vi "Orbitron2Websdr_MainApp.vi"() -> ()   [LabVIEW 2021]
uses:
  Multitrack.llb/Window Rectangle.ctl
  <vilib>/Utility/error.llb/whitespace.ctl
  <vilib>/Utility/error.llb/DialogType.ctl
  <vilib>/Platform/TimedLoop/XDataNode/timing_clust.ctl
  <vilib>/Platform/TimedLoop/XDataNode/nitl_modes.ctl
  <vilib>/Platform/TimedLoop/XDataNode/wakeup.ctl
  <vilib>/Utility/inputDevices.llb/mouseAcquire.vi
  <vilib>/Utility/inputDevices.llb/closeMouse.vi
  <vilib>/Platform/TimedLoop/XDataNode/XDataNode.xnode
  <vilib>/Platform/TimedLoop/XDataNode/XDNodeRunTimeDep.lvlib
  <vilib>/Platform/browser.llb/Open URL in Default Browser (string).vi
panel:
  out "error out 3":errorcluster
  out "error out 2":errorcluster
  out "path 3":path
  in  "Tab Control":T1(tab)
  out "Click":bool
  in  "Lisa":string
  in  "load":bool
  in  "preferences":bool
  in  "cw":bool
  in  "WebPages":u16(ring)=2 items=["IJsselstein, the Netherlands, JO22MA62KJ.", "IS0GRB VHF WebSDR Receiver IS0GRB / south sartinian iland", "Novovoronezh WebSDR WX", "Nürnberg Skyscraper", "Goonhilly Earth Station"]
  in  "Truncate Left digits":i32 caption="kHz"
  in  "processes Box":string(combo)="WebSDR on R3KEE in Novovoronezh - Google Chrome"
  in  "Downlink Freq. Man.":dbl=137100.0 caption="kHz" format="%#_6f"
  in  "ManualLatch":bool
  in  "Radio Mode":bool=TRUE
  in  "Downlink corr.":dbl(knob) scale=-4.0..4.0
  in  "USB":bool
  in  "DeleteWebSDR":bool
  out "Satellite Name":string
  in  "FocusCheck":bool
  in  "Start browser":bool
  in  "Stop_Button":bool
  out "Title 2":string="WebSDR Cat Control"
  in  "FocusWebSDR":bool
  in  "OpenWebSDR":bool
  in  "AddWebSDR":bool
  in  "Stop Cat Control":bool
  in  "Cat Control":bool
  in  "TaskList_Button":bool
  out "Azimuth":string caption="°"
  out "Elevation":string caption="°"
  out "Downlink Freq.":string caption="KHz"
  in  "Type of DN":string
  in  "LSB":bool
  in  "AM":bool
  in  "FM":bool
  in  "EditWebSDR":bool
  out "Mode":string="Radio Manual mode"
  in  "ZoomOut":bool
  in  "ZoomIn":bool
  out "left":i16
  out "right":i16
  out "bottom":i16
  out "top":i16
  out "OverBrowser":bool
  out "MaOps":bool
  in  "Rate 2":i32(slide)=1 min=-10 max=10 scale=-10.0..10.0
  in  "Volume 2":i32(slide)=39 min=0 max=100 scale=0.0..100.0
  in  "TTS Voice":u16(ring)=1 items=["Microsoft Hedda Desktop - German", "Microsoft Zira Desktop - English (United States)"]
  in  "Output Device":u16(ring) items=["Lautsprecher (Realtek(R) Audio)", "CABLE Input (VB-Audio Virtual Cable)"]
  in  "Path of the webbrowser to start WebSDR":path=path "C:/Program Files/Google/Chrome/Application/chrome.exe"
  in  "goback_button":bool
  in  "Cancel Edit 2":bool
  out "data":string caption="DDE Message"
  in  "Sampling interval":u32=1000 caption="[ms]"
  in  "Load_button":bool
  in  "Cancel load":bool
  in  "Load controlfile":path=path "C:/Users/Setup/Documents/LabVIEW 2021"
  in  "Downlink corr.":string="0,000000"
  in  "Title":string="Add a new WebSDR database item"
  in  "Cancel Edit":bool
  in  "Edit_Button":bool
  in  "WebSDR Location / Name":string="Novovoronezh WebSDR WX"
  in  "Cancel Add":bool
  in  "Add_Button":bool
  in  "WebSDR URL":string="http://websdr.vrn.ru:8901/"
  in  "Window title":string="WebSDR on R3KEE in Novovoronezh - Google Chrome"
  in  "Truncate digits":string="2"
  out "Title 3":string="WebSDR Cat Control"
  in  "WebSDRDB":string[][](array[string])=[["IJsselstein, the Netherlands, JO22MA62KJ.", "WebSDR on Gerbrandy Tower in IJsselstein, NL - Google Chrome", "http://websdr.pi1utr.ampr.org:8901/", "0"], ["IS0GRB VHF WebSDR Receiver IS0GRB / south sartinian iland", "IS0GRB VHF WebSDR Receiver - Google Chrome", "http://websdr.is0grb.it:8902/", "2"], ["Novovoronezh WebSDR WX", "WebSDR on R3KEE in Novovoronezh - Google Chrome", "http://websdr.vrn.ru:8901/", "2"]]
  in  "Numeric":i32
  out "error out":errorcluster={"status"=FALSE, "code"=0, "source"="Get Window ID.vi"}
  out "Active Processses":string
  out "standard error":string
  out "standard output":string
  out "window rect 2":T2={"left"=-5, "top"=-564, "right"=1089, "bottom"=-2}
  in  "window names":string[](array[string])=["Orbitron 3.71", "WebSDR on R3KEE in Novovoronezh - Google Chrome", "Mydde", "RX-SSTV", "Task-Manager", "Einstellungen", "Einstellungen", "VIPM Service", "Microsoft Text Input Application", "Mail", "Posteingang – Hotmail ?- Mail", "Orbitron2Websdr_Win10Build", "RX-SSTV", "Program Manager", "LabVIEW"]
  in  "kill":bool
  in  "StopCatProgramatically":bool
  out "shutdown in":bool
  in  "iterCompleted":bool
  in  "slave4Killed":bool
  in  "slave3Killed":bool
  in  "slave1Killed":bool
  out "Elapsed Time (s)":dbl=3.000234603881836
  out "path 2":path
  out "path 4":path=path "C:/Users/Setup/Documents/LabVIEW 2021/Orbitron2Websdr_MainApp_20032021.ctr"
  out "path":path=path "C:/Users/Setup/Documents/LabVIEW 2021/Orbitron2Websdr_MainApp_20032021.ctr"
  out "concatenated string":string="Orbitron2Websdr_MainApp_20032021\\"
  out "string":string="C:\\Users\\Setup\\Documents\\LabVIEW 2021\\Orbitron2Websdr_MainApp_20032021.ctr"
  out "Parent Directory (+ Relative)":path=path "C:/Users/Setup/Documents/LabVIEW 2021"
  in  "dont write":bool
  in  "Interrupt":bool
  in  "AppName":string="WebSDR1"
  # "For Orbitron 3.71 MyDDE-Driver"
  # "To start WebSDR, you need a Webbrowser. We had good experiences using Firefox, so we selected Firefox as the default browser. If you want to start your WebSDR sessions with another browser,just select the executable of your preferred browser here:"
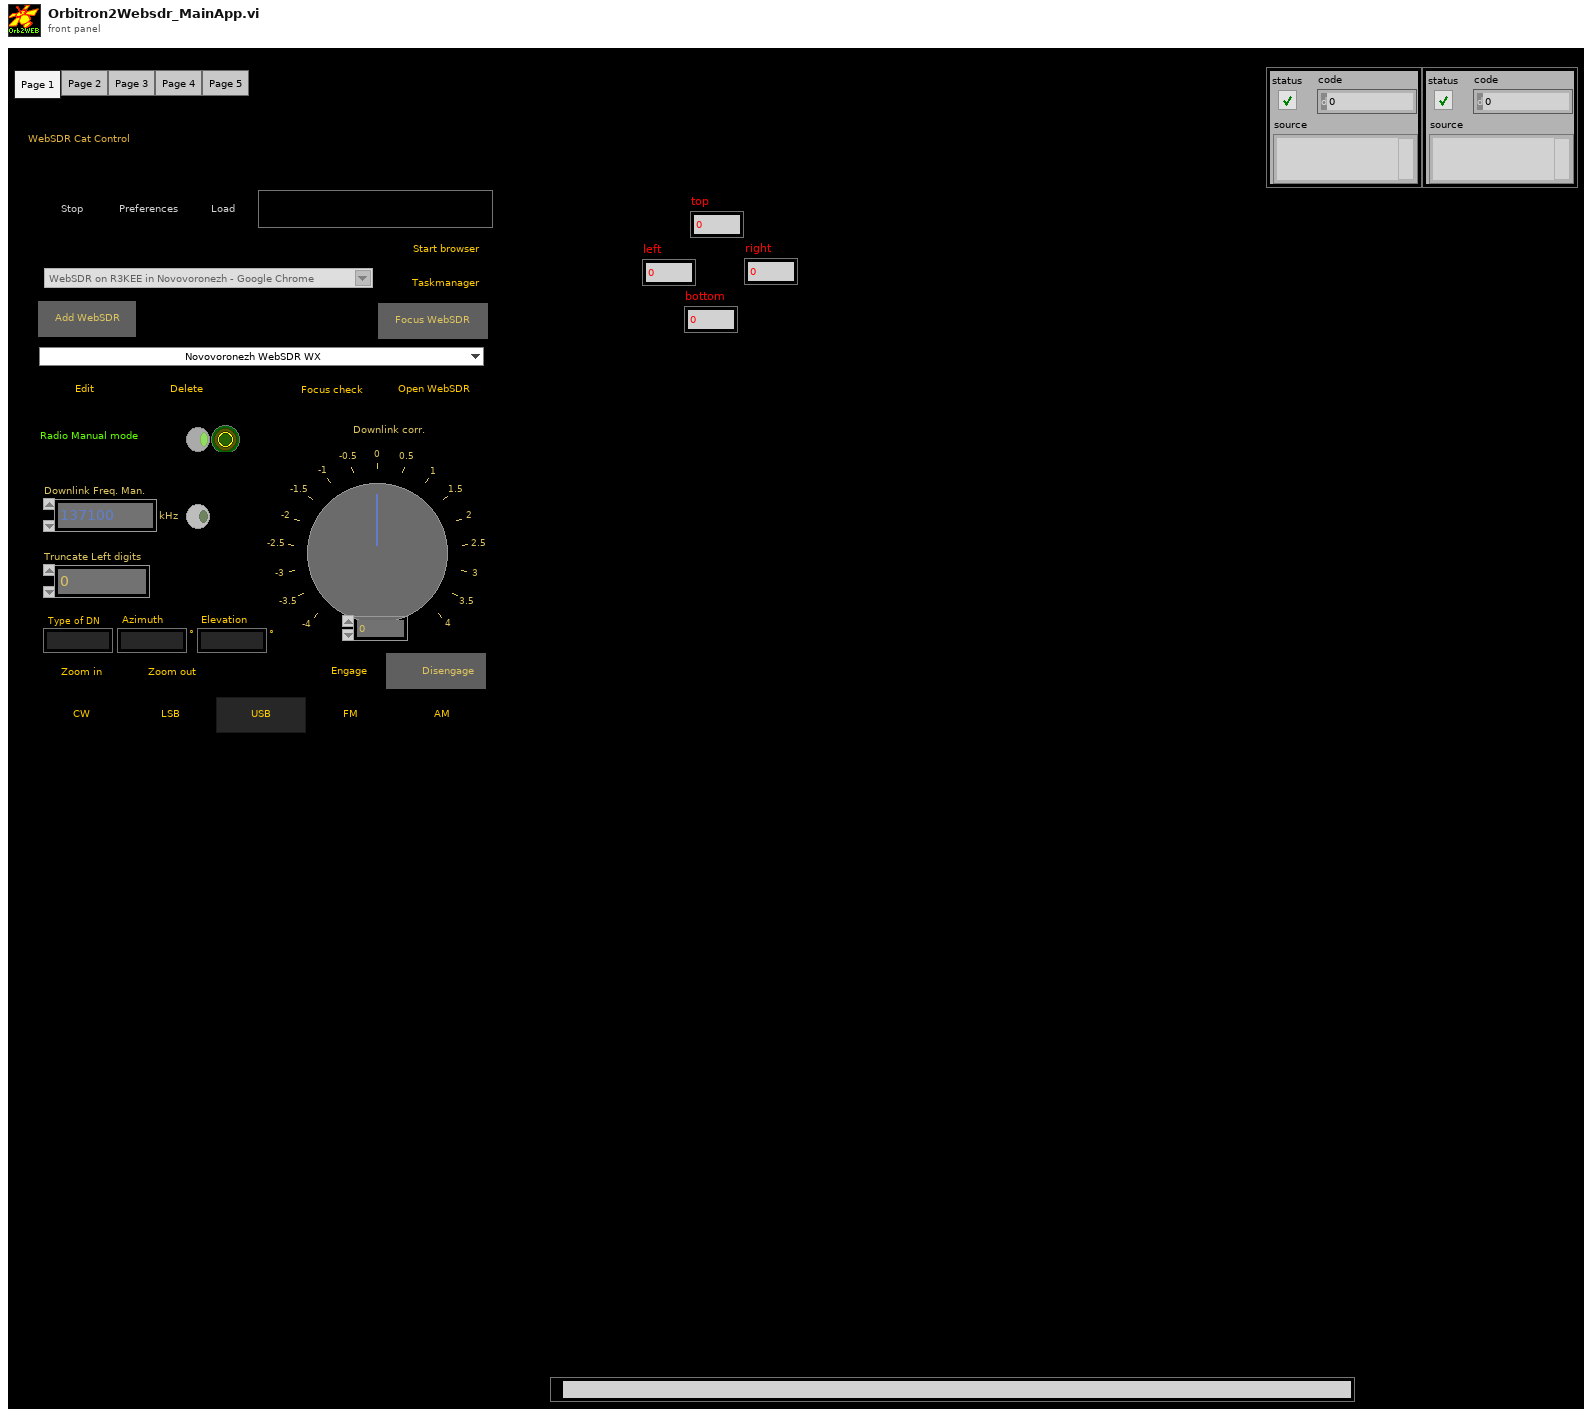
[diagram p1: front panel]
types:
  T1 = enum32{"Page 1", "Page 2", "Page 3", "Page 4", "Page 5"}
  T2 = typedef "Window Rectangle.ctl" = cluster{"left":i16, "top":i16, "right":i16, "bottom":i16}
  T3 = cluster{"Horizontal":i32, "Vertical":i32, "Scrolling":i32}
  T4 = cluster{"button 1":bool, "button 2":bool, "button 3":bool, "button 4":bool}
  T5 = typedef "DialogType.ctl" = u16
  T6 = enum8{"Enabled", "Disabled", "Disabled and Grayed Out"}
  T7 = enum16{"Get Number of Tasks", "Get Window Info", "Get Window Names"}
  T8 = cluster{"number of windows":i32, "total names length":u32, "number of tasks found":i32, "window handles":u32[], "process ID":u32}
  T9 = typedef "Window Refnum" = refnum<k1>
  T10 = typedef "XDNodeRunTimeDep.lvlib/timing_clust.ctl" = cluster{"Expected End [f-1]":u64, "Actual End [f-1]":u64, "Finished Late? [f-1]":bool, "Expected End [i-1]":u64, "Actual End [i-1]":u64, "Finished Late? [i-1]":bool, "Expected Start [i]":u64, "Actual Start [i]":u64, "Expected Start [f]":u64, "Actual Start [f]":u64, "Source Name":string, "Structure Name":string, "Period":i64, "Deadline":i64, "Offset":i64, "Start":i64, "Priority":i32, "Timeout":i32, "Mode":T11, "Wakeup Reason":T12, "Error":errorcluster, "Source Type":string, "Secondary Source Type":string, "Global End Time":u64, "Global Start Time":u64, "Frame Duration":u64, "Iteration Duration":u64, "Assigned CPU":i32, "I/O Scan Engine Mode":u32}
  T11 = typedef "XDNodeRunTimeDep.lvlib/nitl_modes.ctl" = enum32{"No Change", "Process missed periods, maintain original phase", "Discard missed periods, maintain original phase", "Process missed periods, ignore original phase", "Discard missed periods, ignore original phase"}
  T12 = typedef "XDNodeRunTimeDep.lvlib/wakeup.ctl" = enum32{"Normal", "Aborted", "Asynchronous wakeup", "Timing source error", "Timed loop error", "Timeout"}
  T13 = typedef "whitespace.ctl" = u16
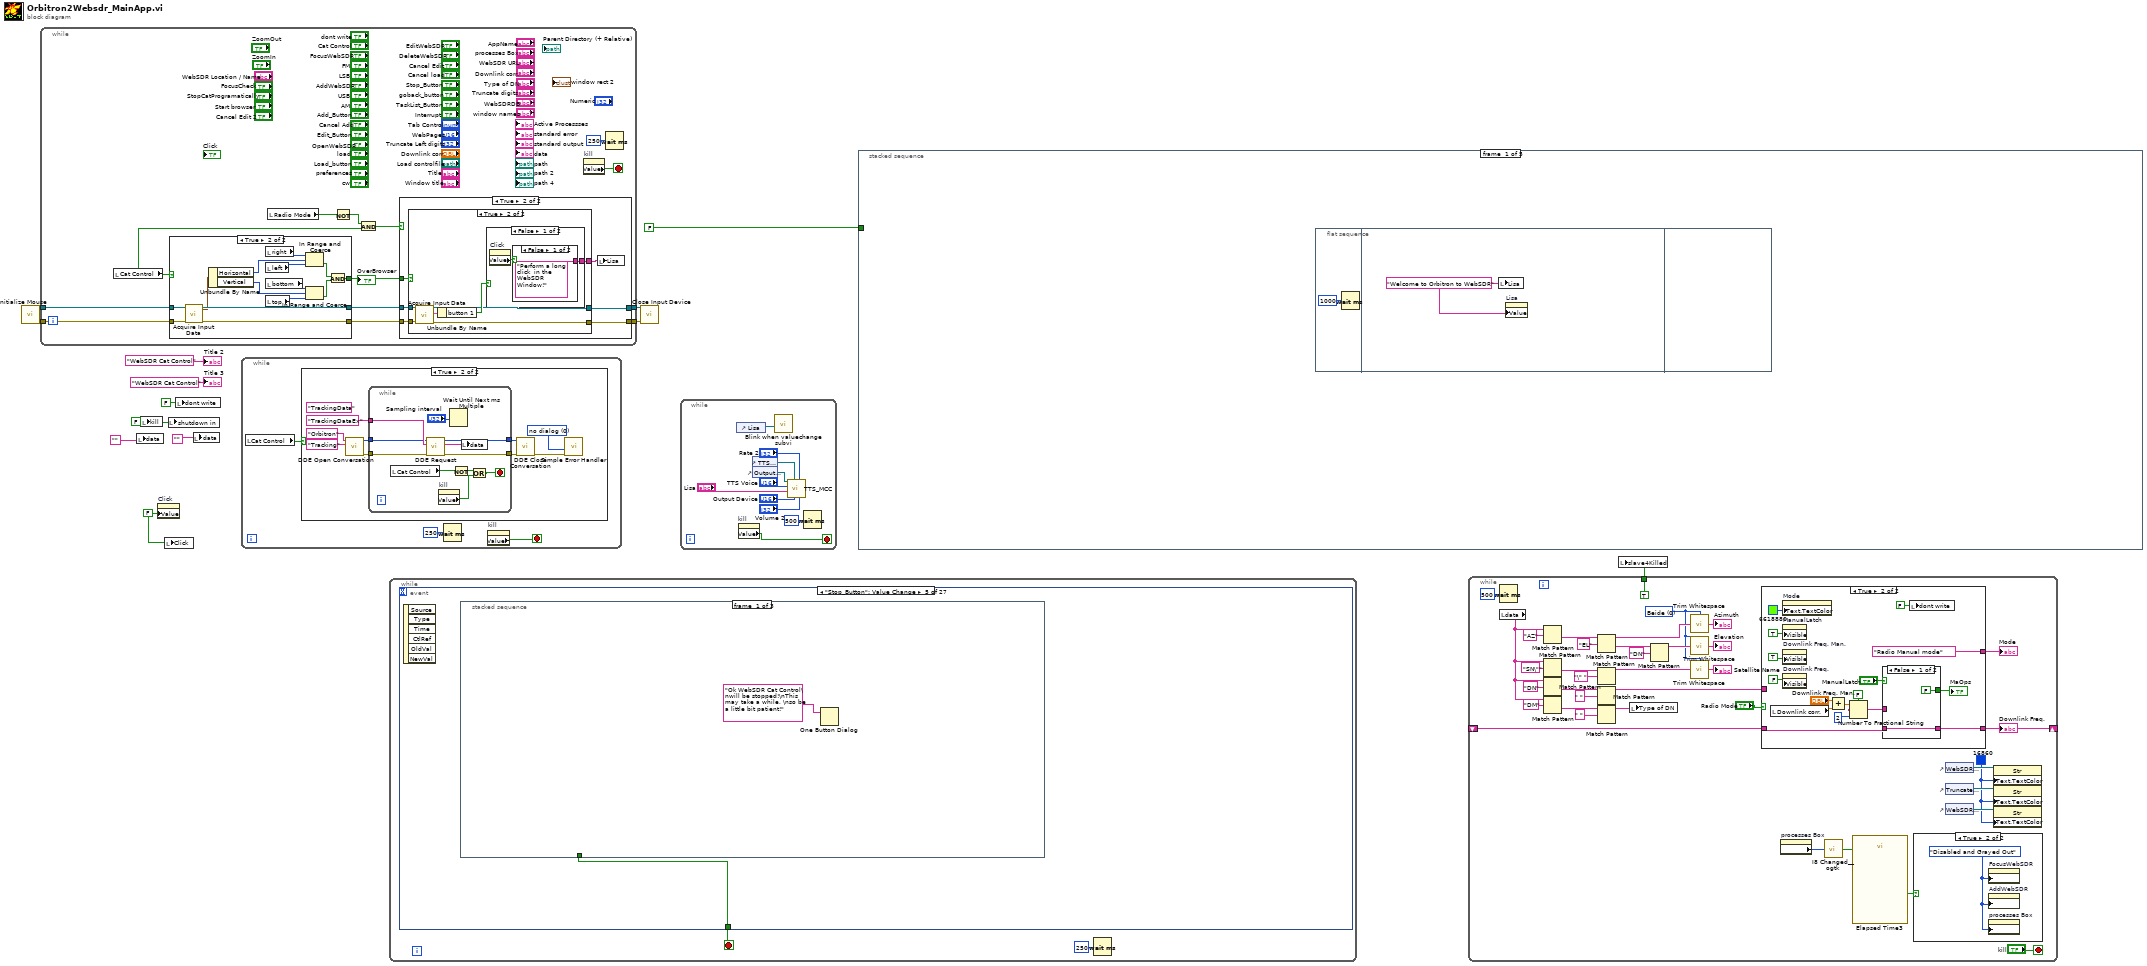
[diagram p0: block diagram]
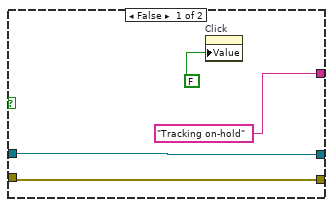
[diagram p3: hidden frame]
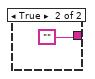
[diagram p4: hidden frame]
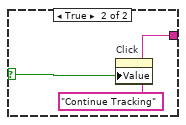
[diagram p5: hidden frame]
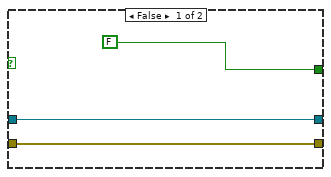
[diagram p6: hidden frame]
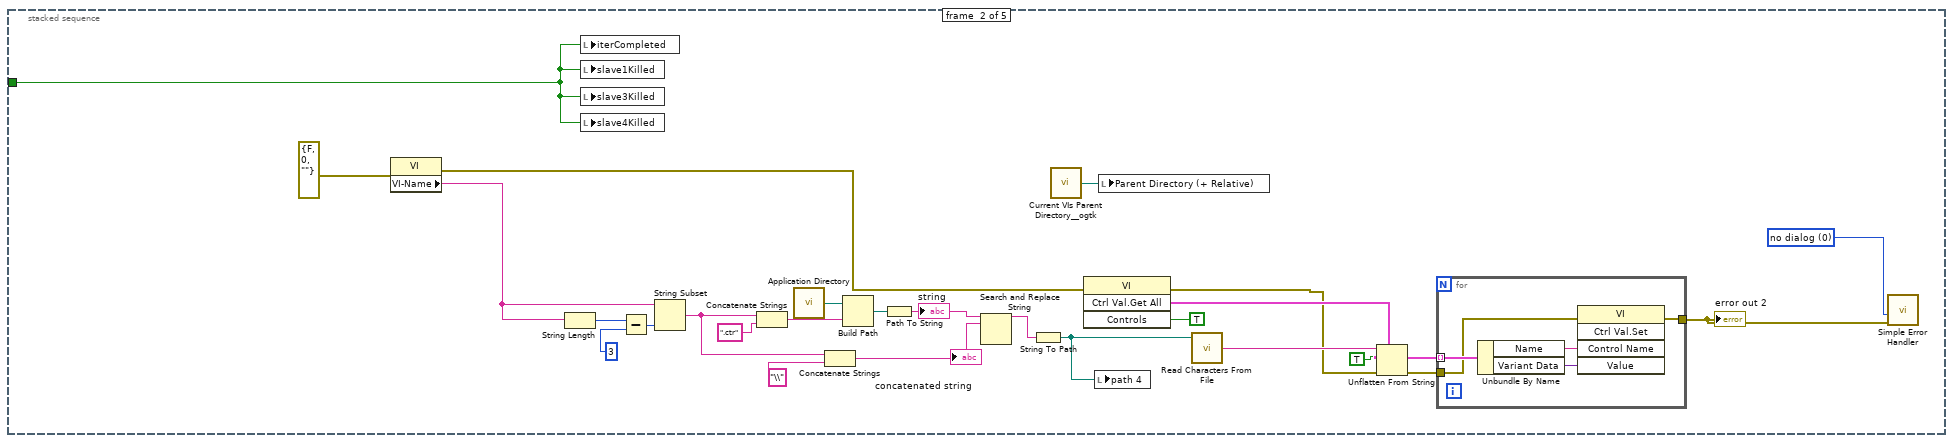
[diagram p8: hidden frame]
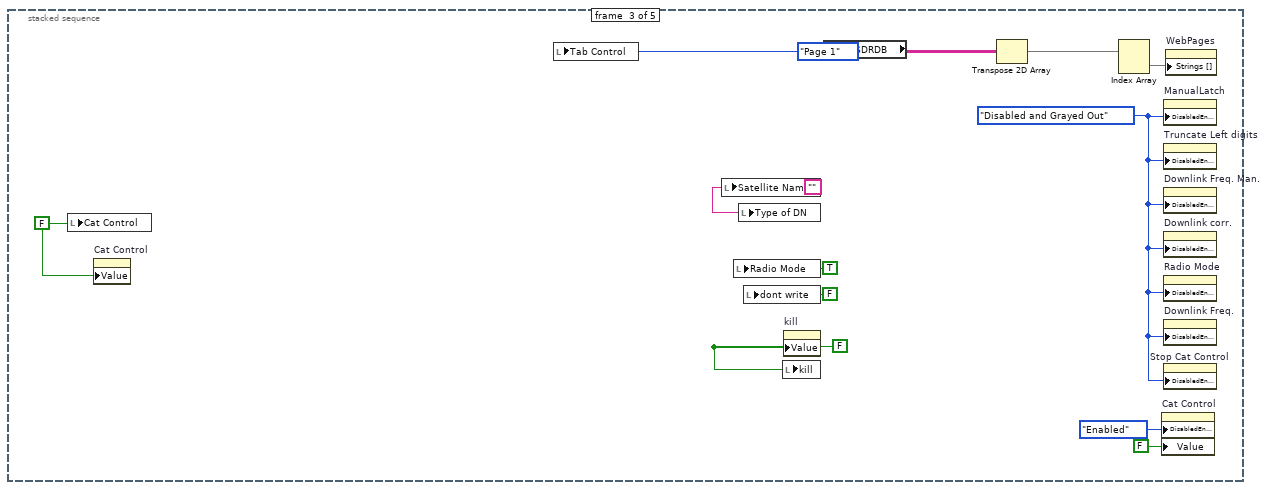
[diagram p9: hidden frame]
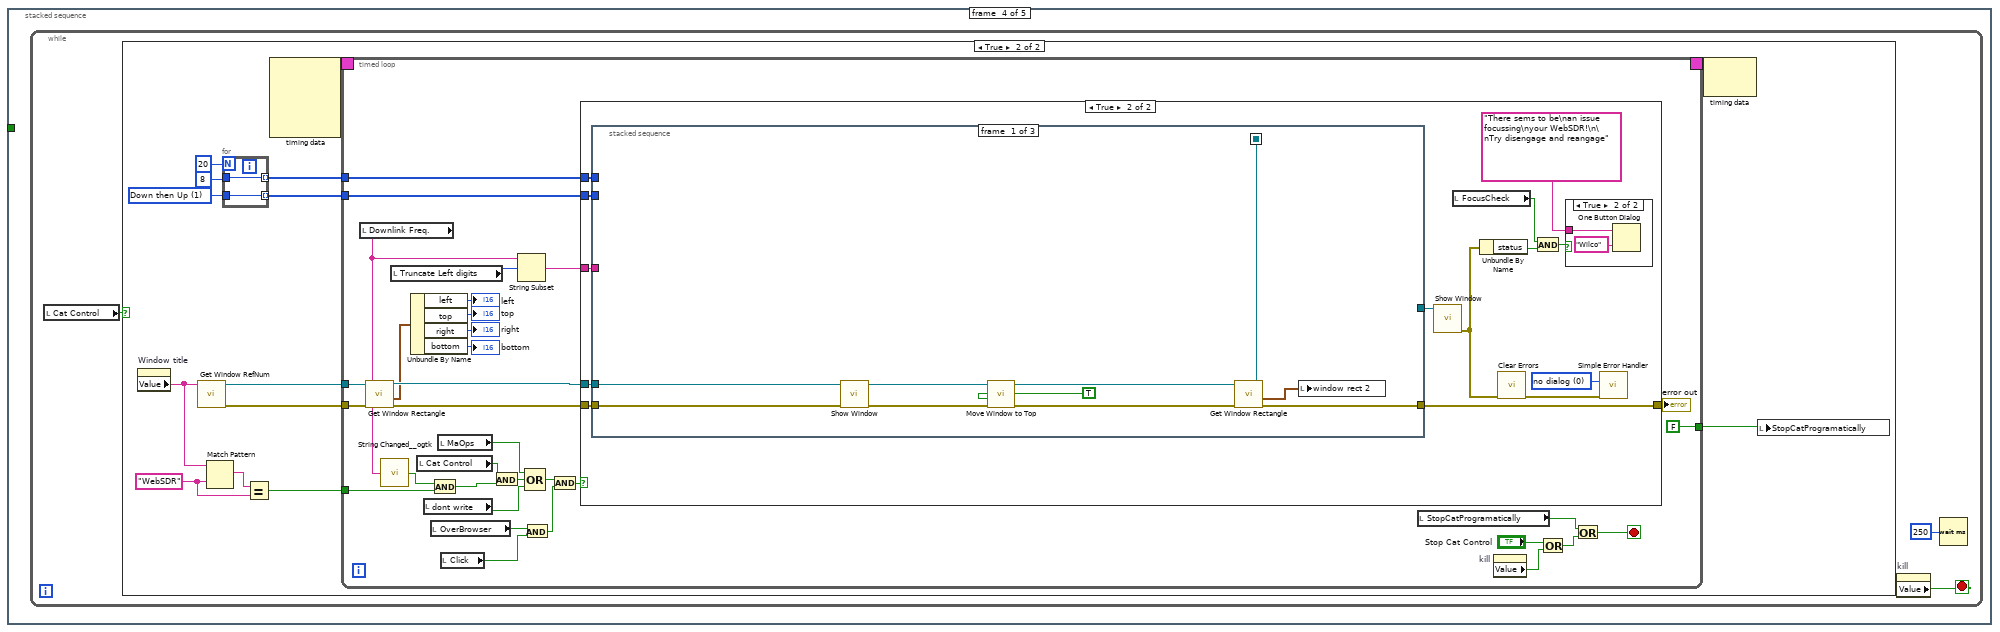
[diagram p10: hidden frame]
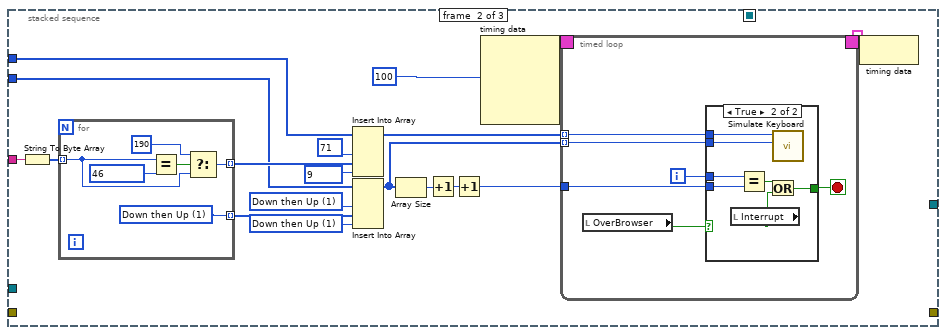
[diagram p14: hidden frame]
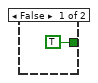
[diagram p15: hidden frame]
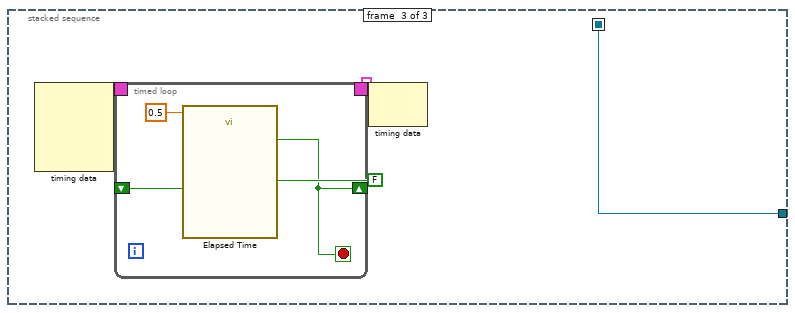
[diagram p16: hidden frame]
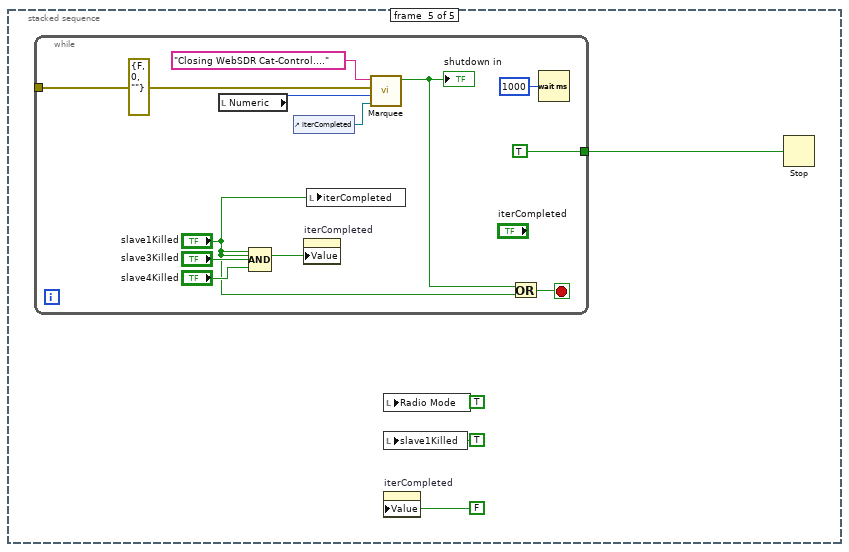
[diagram p17: hidden frame]
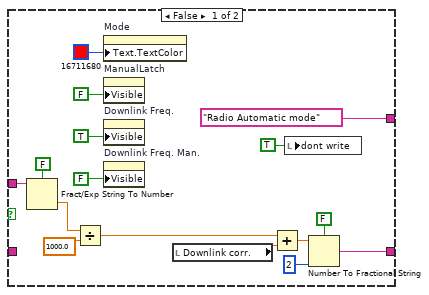
[diagram p19: hidden frame]
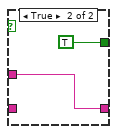
[diagram p20: hidden frame]
diagram:
  w1 = FALSE ("Click")
  w11 = FALSE ("kill")
  n1 = call <vilib>:"Initialize Mouse.vi"() -> ("error out"=w4:errorcluster, "device ID"=w5:refnum<k1>)  [unwired: 10 in]
  n2 = while {
    tunnel: w5 -> [w24]
    tunnel: w4 -> [w23]
    tunnel: [w15] -> w3
    tunnel: [w14] -> w2
    stop <- w26 stop-if-true
    n3 = local read "Cat Control"() -> (w22:bool)
    n4 = case shown="True" w22 {
      tunnel: w24 -> [w53 w68]
      tunnel: w23 -> [w52 w67]
      tunnel: [w53 w66] -> w16
      tunnel: [w52 w65] -> w17
      tunnel: [FALSE w59] -> w20
      frame False {
      }
      frame True {
        n5 = call-poly <vilib>:"Acquire Input Data.vi"("device ID"=w68, "error in (no error)"=w67) -> ("device ID"=w66:refnum<k1>, "axis info"=w64:T3, "error out"=w65:errorcluster)  [unwired: 14 in, 1 out]
        n6 = Unbundle By Name(w64) -> ("Horizontal"=w63:i32, "Vertical"=w62:i32)
        n7 = local read "right"() -> (w56:i16)
        n8 = local read "left"() -> (w55:i16)
        n9 = local read "bottom"() -> (w58:i16)
        n10 = local read "top"() -> (w57:i16)
        n11 = In Range and Coerce(upper limit=w56, x=w63, lower limit=w55) -> (In Range?=w61:bool)  [unwired: 1 out]
        n12 = In Range and Coerce(upper limit=w58, x=w62, lower limit=w57) -> (In Range?=w60:bool)  [unwired: 1 out]
        n13 = And(x=w61, y=w60) -> (x .and. y?=w59:bool)
      }
    }
    "OverBrowser" <- w20
    n14 = local read "Radio Mode"() -> (w19:bool)
    n15 = Not(x=w19) -> (.not. x?=w18:bool)
    n16 = And(x=w18, y=w22) -> (x .and. y?=w21:bool)
    n17 = case shown="True" w21 {
      tunnel: w20 -> [_ w34]
      tunnel: w17 -> [w27 w32]
      tunnel: w16 -> [w28 w33]
      tunnel: [w28 w31] -> w15
      tunnel: [w27 w30] -> w14
      frame False {
      }
      frame True {
        n18 = case shown="True" w34 {
          tunnel: ["Tracking on-hold" ("Lisa 2") w45] -> w29
          tunnel: w33 -> [w37 w44]
          tunnel: w32 -> [w36 w43]
          tunnel: [w37 w40] -> w31
          tunnel: [w36 w39] -> w30
          frame False {
            n19 = property on="Click" class="Bool (strict)"("Value"=FALSE) -> ()  [unwired: 2 in, 2 out]
          }
          frame True {
            n20 = call-poly <vilib>:"Acquire Input Data.vi"("device ID"=w44, "error in (no error)"=w43) -> ("device ID"=w40:refnum<k1>, "button info"=w42:T4, "error out"=w39:errorcluster)  [unwired: 14 in, 1 out]
            n21 = Unbundle By Name(w42) -> ("button 1"=w41:bool)
            n22 = case shown="False" w41 {
              selector: w41 -> [_ w50]
              tunnel: [w47 "Continue Tracking"] -> w45
              frame False {
                n23 = property on="Click" class="Bool (strict)"() -> ("Value"=w46:bool)  [unwired: 2 in, 2 out]
                n24 = case shown="False" w46 {
                  tunnel: ["Perform a long click  in the WebSDR Window!" ""] -> w47
                  frame False {
                  }
                  frame True {
                  }
                }
              }
              frame True {
                n25 = property on="Click" class="Bool (strict)"("Value"=w50) -> ()  [unwired: 2 in, 2 out]
              }
            }
          }
        }
        n26 = local write "Lisa"(w29) -> ()
      }
    }
    n27 = property on="kill" class="Bool (strict)"() -> ("Value"=w26:bool)  [unwired: 2 in, 2 out]
    n28 = Wait (ms)(milliseconds to wait=u32 250) -> ()  [unwired: 1 out]
  }
  n29 = local write "data"("") -> ()
  n30 = local write "kill"(w11) -> ()
  n31 = property on="Click" class="Bool (strict)"("Value"=w1) -> ()  [unwired: 2 in, 2 out]
  n32 = local write "Click"(w1) -> ()
  n33 = local write "shutdown in"(w11) -> ()
  n34 = local write "dont write"(FALSE ("dont write")) -> ()
  n35 = local write "data"("") -> ()
  n36 = while {
    stop <- w71 stop-if-true
    n37 = local read "Cat Control"() -> (w70:bool)
    n38 = case shown="True" w70 {
      frame False {
      }
      frame True {
        w72 = T5 0 items=["no dialog", "OK message", "continue or stop message", "OK message + warnings", "continue/stop + warnings"] ("type of dialog (OK msg:1)")
        (unwired) "TrackingData" ("item")
        n39 = call "DDE Open Conversation.vi"("topic"="Tracking" ("Topic"), "service"="Orbitron" ("Service")) -> ("error out"=w77:errorcluster, "conversation refnum"=w78:u32)  [unwired: 6 in]
        n40 = while {
          tunnel: w78 -> [w90]
          tunnel: w77 -> [w89]
          tunnel: "TrackingDataEx" ("item") -> [w91]
          tunnel: [w88] -> w76
          tunnel: [w87] -> w75
          stop <- w82 stop-if-true
          n41 = local read "Cat Control"() -> (w85:bool)
          n42 = call "DDE Request.vi"("error in (no error)"=w89, "item"=w91, "conversation refnum in"=w90) -> ("error out"=w87:errorcluster, "data"=w84:string, "conversation refnum out"=w88:u32)  [unwired: 4 in]
          n43 = property on="kill" class="Bool (strict)"() -> ("Value"=w81:bool)  [unwired: 2 in, 2 out]
          n44 = Wait Until Next ms Multiple(millisecond multiple="Sampling interval") -> ()  [unwired: 1 out]
          n45 = Not(x=w85) -> (.not. x?=w83:bool)
          n46 = local write "data"(w84) -> ()
          n47 = Or(x=w83, y=w81) -> (x .or. y?=w82:bool)
        }
        n48 = call "DDE Close Conversation.vi"("error in (no error)"=w75, "conversation refnum"=w76) -> ("error out"=w73:errorcluster)  [unwired: 7 in]
        n49 = call <vilib>:"Simple Error Handler.vi"("type of dialog (OK msg:1)"=w72, "error in (no error)"=w73) -> ()  [unwired: 3 in, 5 out]
      }
    }
    n50 = Wait (ms)(milliseconds to wait=u32 250) -> ()  [unwired: 1 out]
    n51 = property on="kill" class="Bool (strict)"() -> ("Value"=w71:bool)  [unwired: 2 in, 2 out]
  }
  n52 = while {
    stop <- w93 stop-if-true
    n53 = event shown="[4] \"Stop_Button\": Value Change" {
      selector: _ -> [_ _ _ _ _ _ _ _ _ _ _ _ _ _ _ _ _ _ _ _ _ _ _ _ _ _ _]
      dyn-events: _ -> [_ _ _ _ _ _ _ _ _ _ _ _ _ _ _ _ _ _ _ _ _ _ _ _ _ _ _]
      timeout: _ -> [_ _ _ _ _ _ _ _ _ _ _ _ _ _ _ _ _ _ _ _ _ _ _ _ _ _ _]
      tunnel: [_ _ _ _ w131 w181 _ _ _ _ _ _ _ _ _ _ _ _ _ _ _ _ _ _ _ _ _] -> w93
      event Timeout {
        n54 = event-data() -> ()  [unwired: 1 in, 3 out]
      }
      event "TaskList_Button": Value Change {
        n55 = event-data() -> ()  [unwired: 1 in, 6 out]
        n56 = stacked-sequence {
          frame #0 {
            n57 = call "WinUtil Master.vi"("function"=T7."Get Window Info") -> ("window enumeration info out"=w98:T8)  [unwired: 4 in, 2 out]
            n58 = call "WinUtil Master.vi"("window enumeration info in"=w98, "function"=T7."Get Window Names") -> ("window names"=w95:string[])  [unwired: 3 in, 2 out]
            n59 = property on="processes Box" class="CmbBox"("DisabledEnum"=T6."Enabled" ("Disabled")) -> ()  [unwired: 2 in, 2 out]
            n60 = control-ref of="processes Box"() -> (w99:refnum<vi>)
            n61 = property on="Property Node" class="CmbBox"(reference=w99, "Strings[]"=w95) -> ()  [unwired: 1 in, 2 out]
            n62 = property on="window names" class="Arr (strict)"("Value"=w95) -> ()  [unwired: 2 in, 2 out]
            n63 = local write "window names"(w95) -> ()
          }
        }
      }
      event "processes Box": Value Change {
        w101 = "WebSDR" ("Such-String")
        w104 = T6."Enabled" ("Disabled")
        n64 = event-data() -> ("NewVal"=w103:string)  [unwired: 1 in, 5 out]
        n65 = Match Pattern(string=w103, regular expression=w101) -> (match substring=w102:string)  [unwired: 1 in, 3 out]
        n66 = property on="AddWebSDR" class="Bool"("DisabledEnum"=w104) -> ()  [unwired: 2 in, 2 out]
        n67 = property on="FocusWebSDR" class="Bool"("DisabledEnum"=w104) -> ()  [unwired: 2 in, 2 out]
        n68 = Equal?(x=w102, y=w101) -> (x = y?=w100:bool)
        n69 = case shown="False" w100 {
          tunnel: w103 -> [w105 w111]
          frame False {
            n70 = Two Button Dialog(message="The selected application does\nnot seem to be related to WebSDR!\n\nAre you sure?", 1:"No, I better go verify..." ("F button name (\"Cancel\")"), 2:"Yes" ("T button name (\"OK\")")) -> (T button?=w106:bool)
            n71 = case shown="True" w106 {
              tunnel: w105 -> [_ w110]
              frame False {
              }
              frame True {
                n72 = property on="Window title" class="Str"("Value"=w110) -> ()  [unwired: 2 in, 2 out]
              }
            }
          }
          frame True {
            n73 = property on="Window title" class="Str"("Value"=w111) -> ()  [unwired: 2 in, 2 out]
          }
        }
      }
      event "Cat Control": Value Change {
        n74 = event-data() -> ()  [unwired: 1 in, 6 out]
        n75 = stacked-sequence {
          seq-local: [_ _ w122 _] -> [_ _ _ w128]
          frame #0 {
            w112 = T6."Enabled" ("Disabled")
            n76 = property on="ManualLatch" class="Bool"("DisabledEnum"=w112) -> ()  [unwired: 2 in, 2 out]
            n77 = property on="Truncate Left digits" class="DigNum (strict)"("DisabledEnum"=w112) -> ()  [unwired: 2 in, 2 out]
            n78 = property on="Downlink Freq. Man." class="DigNum (strict)"("DisabledEnum"=w112) -> ()  [unwired: 2 in, 2 out]
            n79 = property on="Downlink corr." class="Knob (strict)"("DisabledEnum"=w112) -> ()  [unwired: 2 in, 2 out]
            n80 = property on="Radio Mode" class="Bool (strict)"("DisabledEnum"=w112) -> ()  [unwired: 2 in, 2 out]
            n81 = property on="Downlink Freq." class="Str"("DisabledEnum"=w112) -> ()  [unwired: 2 in, 2 out]
            n82 = property on="Cat Control" class="Bool (strict)"("DisabledEnum"=T6."Disabled and Grayed Out" ("Disabled")) -> ()  [unwired: 2 in, 2 out]
            n83 = property on="Stop Cat Control" class="Bool"("DisabledEnum"=T6."Enabled" ("Disabled")) -> ()  [unwired: 2 in, 2 out]
          }
          frame #1 {
            n84 = while {
              shift-right: [FALSE] -> _
              shift-left: TRUE -> [w117]
              stop <- w119 stop-if-true
              n85 = call "Elapsed Time2"("Time Target (s)"=5.0, "Reset"=w117) -> ("Elapsed Time (s)"=→"Elapsed Time (s)":dbl, "Time has Elapsed"=w119:bool)  [unwired: 10 in, 6 out]
            }
          }
          frame #2 {
            n86 = property on="data" class="Str"() -> ("Value"=w121:string)  [unwired: 2 in, 2 out]
            n87 = Match Pattern(string=w121, regular expression="SN" ("Regulärer Ausdruck")) -> (offset past match=w124:i32)  [unwired: 1 in, 3 out]
            n88 = Equal?(x=w124, y=-1) -> (x = y?=w122:bool)
            n89 = case shown="True" w122 {
              frame False {
              }
              frame True {
                n90 = One Button Dialog(message="Error:\nPlease disengage and verify that\nOrbitron MyDDE- Driver is up and\nrunning!", button name ("OK")="Oh yeah: sure!") -> ()  [unwired: 1 out]
              }
            }
          }
          frame #3 {
            n91 = case shown="False" w128 {
              frame False {
                n92 = local write "Lisa"("Success: DDE Connection Established!") -> ()
                n93 = call "Display Message to User2"("Message"="Success: MyDDE Connection Established!\n\nSet focus to the WebSDR-site, by bringing it to front most and klick into the frequency Controlbox of the site.") -> ()  [unwired: 9 in, 2 out]
              }
              frame True {
              }
            }
          }
        }
      }
      event "Stop_Button": Value Change {
        n94 = event-data() -> ()  [unwired: 1 in, 6 out]
        n95 = stacked-sequence {
          tunnel: [_ _ w180] -> w131
          frame #0 {
            n96 = One Button Dialog(message="Ok WebSDR Cat Control\nwill be stopped!\nThis may take a while, \nso be a little bit patient!") -> ()  [unwired: 1 in, 1 out]
          }
          frame #1 {
            w141 = "websdrOrbitron" ("regular expression")
            n97 = property class="VI"() -> ("VI-Name"=w151:string)  [unwired: 2 in, 2 out]
            n98 = call "Current VIs Parent Directory__ogtk.vi"() -> ("Parent Directory (+ Relative)"=w135:path)  [unwired: 5 in]
            n99 = String Length(string=w151) -> (length=w149:i32)
            n100 = Subtract(x=w149, y=3) -> (x-y=w150:i32)
            n101 = String Subset(string=w151, length (rest)=w150) -> (substring=w168:string)  [unwired: 1 in]
            n102 = Concatenate Strings(w168, "*" ("string")) -> (w166:string)
            n103 = List Folder(path=w135, pattern=w166) -> (filenames=w167:string[])  [unwired: 2 in, 3 out]
            n104 = for {
              tunnel: w167 -> [w169] mode=indexing
              tunnel: w141 -> [w172]
              tunnel: [w171] -> w157 mode=indexing
              tunnel: [w169] -> _ mode=indexing
              n105 = Match Pattern(string=w169, regular expression=w172) -> (after substring=w170:string)  [unwired: 1 in, 3 out]
              n106 = Decimal String To Number(string=w170) -> (number=w171:i32)  [unwired: 2 in, 1 out]
            }
            n107 = Concatenate Strings(w168, ".ctr" ("String")) -> (w165:string)
            n108 = Build Path(base path=w135, name or relative path=w165) -> (appended path=w145:path)
            n109 = Array Max & Min(array=w157) -> (max value=w164:i32)  [unwired: 3 out]
            n110 = Concatenate Strings(w151, "\\" ("string")) -> (w148:string)
            n111 = Path To String(path=w145) -> (string=w146:string)
            n112 = Increment(x=w164) -> (x+1=w156:i32)
            n113 = Search and Replace String(input string=w146, search string=w148) -> (result string=w147:string)  [unwired: 6 in, 3 out]
            n114 = Format Value(format string="%03d", value (0)=w156) -> (output string=w155:string)  [unwired: 1 in]
            n115 = String To Path(string=w147) -> (path=w152:path)
            n116 = local write "path"(w152) -> ()
            n117 = Concatenate Strings(w141, w155) -> (w163:string)
            n118 = Concatenate Strings(w163, ".ctr" ("String")) -> (w158:string)
            n119 = invoke class="VI" method="Ctrl Val.Get All"("Controls"=TRUE ("controls")) -> ("Get All Control Values Variant"=w153:cluster{"Name":string, "Variant Data":variant}[])  [unwired: 3 in, 3 out]
            n120 = Build Path(base path=w135, name or relative path=w158) -> (appended path=w162:path)
            n121 = Concatenate Strings(w163, "\\" ("string")) -> (w159:string)
            n122 = Path To String(path=w162) -> (string=w161:string)
            n123 = Search and Replace String(input string=w161, search string=w159) -> (result string=w160:string)  [unwired: 6 in, 3 out]
            n124 = String To Path(string=w160) -> (path=w134:path)
            n125 = Flatten To String(anything=w153, prepend array or string size? (T)=TRUE) -> (data string=w154:string)  [unwired: 2 in, 2 out]
            n126 = stacked-sequence {
              tunnel: w152 -> [_ w175 _ w178 _]
              tunnel: w154 -> [w173 _ _ w177 _]
              tunnel: w134 -> [w174 _ _ _ _]
              frame #0 {
                n127 = call <vilib>:"Write Characters To File.vi"("character string"=w173, "file path (dialog if empty)"=w174) -> ()  [unwired: 3 in, 1 out]
              }
              frame #1 {
                n128 = Delete(path (use dialog)=w175) -> ()  [unwired: 4 in, 3 out]
              }
              frame #2 {
                n129 = Wait (ms)(milliseconds to wait=u32 2000) -> ()  [unwired: 1 out]
              }
              frame #3 {
                n130 = call <vilib>:"Write Characters To File.vi"("character string"=w177, "file path (dialog if empty)"=w178) -> ()  [unwired: 3 in, 1 out]
              }
              frame #4 {
                n131 = Wait (ms)(milliseconds to wait=u32 2000) -> ()  [unwired: 1 out]
              }
            }
          }
          frame #2 {
            w180 = TRUE ("kill")
            n132 = property on="kill" class="Bool (strict)"("Value"=w180) -> ()  [unwired: 2 in, 2 out]
          }
        }
      }
      event Panel Close? {
        n133 = event-data() -> ()  [unwired: 1 in, 4 out]
        n134 = stacked-sequence {
          tunnel: [_ _ _ w232] -> w181
          frame #0 {
            n135 = One Button Dialog(message="Ok WebSDR Cat Control\nwill be stoped!\nThis may take a while, \nso be a little bit patient!") -> ()  [unwired: 1 in, 1 out]
          }
          frame #1 {
            w190 = "websdrOrbitron" ("regular expression")
            n136 = property class="VI"() -> ("VI-Name"=w200:string)  [unwired: 2 in, 2 out]
            n137 = call "Current VIs Parent Directory__ogtk.vi"() -> ("Parent Directory (+ Relative)"=w212:path)  [unwired: 5 in]
            n138 = String Length(string=w200) -> (length=w198:i32)
            n139 = Subtract(x=w198, y=3) -> (x-y=w199:i32)
            n140 = String Subset(string=w200, length (rest)=w199) -> (substring=w218:string)  [unwired: 1 in]
            n141 = Concatenate Strings(w218, "*" ("string")) -> (w216:string)
            n142 = List Folder(path=w212, pattern=w216) -> (filenames=w217:string[])  [unwired: 2 in, 3 out]
            n143 = for {
              tunnel: w217 -> [w219] mode=indexing
              tunnel: w190 -> [w222]
              tunnel: [w221] -> w206 mode=indexing
              tunnel: [w219] -> _ mode=indexing
              n144 = Match Pattern(string=w219, regular expression=w222) -> (after substring=w220:string)  [unwired: 1 in, 3 out]
              n145 = Decimal String To Number(string=w220) -> (number=w221:i32)  [unwired: 2 in, 1 out]
            }
            n146 = Concatenate Strings(w218, ".ctr" ("String")) -> (w215:string)
            n147 = Build Path(base path=w212, name or relative path=w215) -> (appended path=w194:path)
            n148 = Array Max & Min(array=w206) -> (max value=w214:i32)  [unwired: 3 out]
            n149 = Concatenate Strings(w200, "\\" ("string")) -> (w197:string)
            n150 = Path To String(path=w194) -> (string=w195:string)
            n151 = Increment(x=w214) -> (x+1=w205:i32)
            n152 = Search and Replace String(input string=w195, search string=w197) -> (result string=w196:string)  [unwired: 6 in, 3 out]
            n153 = Format Value(format string="%03d", value (0)=w205) -> (output string=w204:string)  [unwired: 1 in]
            n154 = String To Path(string=w196) -> (path=w201:path)
            n155 = local write "path"(w201) -> ()
            n156 = Concatenate Strings(w190, w204) -> (w213:string)
            n157 = invoke class="VI" method="Ctrl Val.Get All"("Controls"=TRUE ("controls")) -> ("Get All Control Values Variant"=w202:cluster{"Name":string, "Variant Data":variant}[])  [unwired: 3 in, 3 out]
            n158 = Concatenate Strings(w213, ".ctr" ("String")) -> (w207:string)
            n159 = Build Path(base path=w212, name or relative path=w207) -> (appended path=w211:path)
            n160 = Concatenate Strings(w213, "\\" ("string")) -> (w208:string)
            n161 = Path To String(path=w211) -> (string=w210:string)
            n162 = Search and Replace String(input string=w210, search string=w208) -> (result string=w209:string)  [unwired: 6 in, 3 out]
            n163 = Flatten To String(anything=w202, prepend array or string size? (T)=TRUE) -> (data string=w203:string)  [unwired: 2 in, 2 out]
            n164 = String To Path(string=w209) -> (path=w184:path)
            n165 = stacked-sequence {
              tunnel: w201 -> [_ w227 _ w230 _]
              tunnel: w203 -> [w223 _ _ w229 _]
              tunnel: w184 -> [w224 _ _ _ _]
              frame #0 {
                n166 = call <vilib>:"Write Characters To File.vi"("character string"=w223, "file path (dialog if empty)"=w224) -> ()  [unwired: 3 in, 1 out]
              }
              frame #1 {
                w226 = T5 0 items=["no dialog", "OK message", "continue or stop message", "OK message + warnings", "continue/stop + warnings"] ("type of dialog (OK msg:1)")
                n167 = Delete(path (use dialog)=w227) -> (error out=w225:errorcluster)  [unwired: 4 in, 2 out]
                n168 = call <vilib>:"Simple Error Handler.vi"("type of dialog (OK msg:1)"=w226, "error in (no error)"=w225) -> ()  [unwired: 3 in, 5 out]
              }
              frame #2 {
                n169 = Wait (ms)(milliseconds to wait=u32 4000) -> ()  [unwired: 1 out]
              }
              frame #3 {
                n170 = call <vilib>:"Write Characters To File.vi"("character string"=w229, "file path (dialog if empty)"=w230) -> ()  [unwired: 3 in, 1 out]
              }
              frame #4 {
                n171 = Wait (ms)(milliseconds to wait=u32 2000) -> ()  [unwired: 1 out]
              }
            }
            n172 = local write "path 2"(w184) -> ()
          }
          frame #2 {
          }
          frame #3 {
            w232 = TRUE ("kill")
            n173 = property on="kill" class="Bool (strict)"("Value"=w232) -> ()  [unwired: 2 in, 2 out]
          }
        }
        n174 = event-data("Discard?"=w181) -> ()  [unwired: 1 in, 1 out]
      }
      event "USB": Value Change {
        w238 = "WebSDR" ("Such-String")
        n175 = event-data() -> ()  [unwired: 1 in, 6 out]
        n176 = local read "Window title"() -> (w236:string)
        n177 = call "Get Window RefNum.vi"("window name (\"\")"=w236) -> ("error out"=w233:errorcluster, "window refnum (NaWR)"=w234:T9)  [unwired: 7 in]
        n178 = Match Pattern(string=w236, regular expression=w238) -> (match substring=w237:string)  [unwired: 1 in, 3 out]
        n179 = Equal?(x=w237, y=w238) -> (x = y?=w235:bool)
        n180 = case shown="True" w235 {
          tunnel: w234 -> [_ w243]
          tunnel: w233 -> [_ w242]
          frame False {
          }
          frame True {
            n181 = stacked-sequence {
              tunnel: w243 -> [w250 _]
              tunnel: w242 -> [w249 _]
              tunnel: [w248 _] -> w241
              tunnel: [w247 _] -> w240
              tunnel: [w246 _] -> w239
              frame #0 {
                n182 = call "Show Window.vi"("error in (no error)"=w249, "window refnum (NaWR)"=w250) -> ("error out"=w245:errorcluster, "window refnum out"=w253:T9)  [unwired: 4 in]
                n183 = call "Move Window to Top.vi"("error in (no error)"=w245, "activate? (T)"=TRUE ("activate? (F)"), "window refnum (NaWR)"=w253) -> ("error out"=w244:errorcluster, "window refnum out"=w252:T9)  [unwired: 3 in]
                n184 = call "Get Window Rectangle.vi"("error in (no error)"=w244, "window refnum (NaWR)"=w252) -> ("error out"=w247:errorcluster, "window rect"=w246:T2, "window refnum out"=w248:T9)  [unwired: 3 in]
              }
              frame #1 {
                w254 = u32 1 items=["Down/Press", "Down then Up", "Up/Release"] ("Action")
                n185 = call "Simulate Keyboard.vi"("Action"=w254, "Virtual Key"=u8 85) -> ()  [unwired: 7 in, 1 out]
              }
            }
            n186 = local write "window rect 2"(w239) -> ()
            n187 = call "Show Window.vi"("error in (no error)"=w240, "window refnum (NaWR)"=w241) -> ()  [unwired: 4 in, 2 out]
          }
        }
      }
      event "cw": Value Change {
        w261 = "WebSDR" ("Such-String")
        n188 = event-data() -> ()  [unwired: 1 in, 6 out]
        n189 = local read "Window title"() -> (w259:string)
        n190 = call "Get Window RefNum.vi"("window name (\"\")"=w259) -> ("error out"=w256:errorcluster, "window refnum (NaWR)"=w257:T9)  [unwired: 7 in]
        n191 = Match Pattern(string=w259, regular expression=w261) -> (match substring=w260:string)  [unwired: 1 in, 3 out]
        n192 = Equal?(x=w260, y=w261) -> (x = y?=w258:bool)
        n193 = case shown="True" w258 {
          tunnel: w257 -> [_ w266]
          tunnel: w256 -> [_ w265]
          frame False {
          }
          frame True {
            n194 = stacked-sequence {
              tunnel: w266 -> [w273 _]
              tunnel: w265 -> [w272 _]
              tunnel: [w271 _] -> w264
              tunnel: [w270 _] -> w263
              tunnel: [w269 _] -> w262
              frame #0 {
                n195 = call "Show Window.vi"("error in (no error)"=w272, "window refnum (NaWR)"=w273) -> ("error out"=w268:errorcluster, "window refnum out"=w276:T9)  [unwired: 4 in]
                n196 = call "Move Window to Top.vi"("error in (no error)"=w268, "activate? (T)"=TRUE ("activate? (F)"), "window refnum (NaWR)"=w276) -> ("error out"=w267:errorcluster, "window refnum out"=w275:T9)  [unwired: 3 in]
                n197 = call "Get Window Rectangle.vi"("error in (no error)"=w267, "window refnum (NaWR)"=w275) -> ("error out"=w270:errorcluster, "window rect"=w269:T2, "window refnum out"=w271:T9)  [unwired: 3 in]
              }
              frame #1 {
                w277 = u32 1 items=["Down/Press", "Down then Up", "Up/Release"] ("Action")
                n198 = call "Simulate Keyboard.vi"("Action"=w277, "Virtual Key"=u8 67) -> ()  [unwired: 7 in, 1 out]
              }
            }
            n199 = local write "window rect 2"(w262) -> ()
            n200 = call "Show Window.vi"("error in (no error)"=w263, "window refnum (NaWR)"=w264) -> ()  [unwired: 4 in, 2 out]
          }
        }
      }
      event "LSB": Value Change {
        w284 = "WebSDR" ("Such-String")
        n201 = event-data() -> ()  [unwired: 1 in, 6 out]
        n202 = local read "Window title"() -> (w282:string)
        n203 = call "Get Window RefNum.vi"("window name (\"\")"=w282) -> ("error out"=w279:errorcluster, "window refnum (NaWR)"=w280:T9)  [unwired: 7 in]
        n204 = Match Pattern(string=w282, regular expression=w284) -> (match substring=w283:string)  [unwired: 1 in, 3 out]
        n205 = Equal?(x=w283, y=w284) -> (x = y?=w281:bool)
        n206 = case shown="True" w281 {
          tunnel: w280 -> [_ w289]
          tunnel: w279 -> [_ w288]
          frame False {
          }
          frame True {
            n207 = stacked-sequence {
              tunnel: w289 -> [w296 _]
              tunnel: w288 -> [w295 _]
              tunnel: [w294 _] -> w287
              tunnel: [w293 _] -> w286
              tunnel: [w292 _] -> w285
              frame #0 {
                n208 = call "Show Window.vi"("error in (no error)"=w295, "window refnum (NaWR)"=w296) -> ("error out"=w291:errorcluster, "window refnum out"=w299:T9)  [unwired: 4 in]
                n209 = call "Move Window to Top.vi"("error in (no error)"=w291, "activate? (T)"=TRUE ("activate? (F)"), "window refnum (NaWR)"=w299) -> ("error out"=w290:errorcluster, "window refnum out"=w298:T9)  [unwired: 3 in]
                n210 = call "Get Window Rectangle.vi"("error in (no error)"=w290, "window refnum (NaWR)"=w298) -> ("error out"=w293:errorcluster, "window rect"=w292:T2, "window refnum out"=w294:T9)  [unwired: 3 in]
              }
              frame #1 {
                w300 = u32 1 items=["Down/Press", "Down then Up", "Up/Release"] ("Action")
                n211 = call "Simulate Keyboard.vi"("Action"=w300, "Virtual Key"=u8 76) -> ()  [unwired: 7 in, 1 out]
              }
            }
            n212 = local write "window rect 2"(w285) -> ()
            n213 = call "Show Window.vi"("error in (no error)"=w286, "window refnum (NaWR)"=w287) -> ()  [unwired: 4 in, 2 out]
          }
        }
      }
      event "FM": Value Change {
        w307 = "WebSDR" ("Such-String")
        n214 = event-data() -> ()  [unwired: 1 in, 6 out]
        n215 = local read "Window title"() -> (w305:string)
        n216 = call "Get Window RefNum.vi"("window name (\"\")"=w305) -> ("error out"=w302:errorcluster, "window refnum (NaWR)"=w303:T9)  [unwired: 7 in]
        n217 = Match Pattern(string=w305, regular expression=w307) -> (match substring=w306:string)  [unwired: 1 in, 3 out]
        n218 = Equal?(x=w306, y=w307) -> (x = y?=w304:bool)
        n219 = case shown="True" w304 {
          tunnel: w303 -> [_ w312]
          tunnel: w302 -> [_ w311]
          frame False {
          }
          frame True {
            n220 = stacked-sequence {
              tunnel: w312 -> [w319 _]
              tunnel: w311 -> [w318 _]
              tunnel: [w317 _] -> w310
              tunnel: [w316 _] -> w309
              tunnel: [w315 _] -> w308
              frame #0 {
                n221 = call "Show Window.vi"("error in (no error)"=w318, "window refnum (NaWR)"=w319) -> ("error out"=w314:errorcluster, "window refnum out"=w322:T9)  [unwired: 4 in]
                n222 = call "Move Window to Top.vi"("error in (no error)"=w314, "activate? (T)"=TRUE ("activate? (F)"), "window refnum (NaWR)"=w322) -> ("error out"=w313:errorcluster, "window refnum out"=w321:T9)  [unwired: 3 in]
                n223 = call "Get Window Rectangle.vi"("error in (no error)"=w313, "window refnum (NaWR)"=w321) -> ("error out"=w316:errorcluster, "window rect"=w315:T2, "window refnum out"=w317:T9)  [unwired: 3 in]
              }
              frame #1 {
                w323 = u32 1 items=["Down/Press", "Down then Up", "Up/Release"] ("Action")
                n224 = call "Simulate Keyboard.vi"("Action"=w323, "Virtual Key"=u8 70) -> ()  [unwired: 7 in, 1 out]
              }
            }
            n225 = local write "window rect 2"(w308) -> ()
            n226 = call "Show Window.vi"("error in (no error)"=w309, "window refnum (NaWR)"=w310) -> ()  [unwired: 4 in, 2 out]
          }
        }
      }
      event "AM": Value Change {
        w330 = "WebSDR" ("Such-String")
        n227 = event-data() -> ()  [unwired: 1 in, 6 out]
        n228 = local read "Window title"() -> (w328:string)
        n229 = call "Get Window RefNum.vi"("window name (\"\")"=w328) -> ("error out"=w325:errorcluster, "window refnum (NaWR)"=w326:T9)  [unwired: 7 in]
        n230 = Match Pattern(string=w328, regular expression=w330) -> (match substring=w329:string)  [unwired: 1 in, 3 out]
        n231 = Equal?(x=w329, y=w330) -> (x = y?=w327:bool)
        n232 = case shown="True" w327 {
          tunnel: w326 -> [_ w335]
          tunnel: w325 -> [_ w334]
          frame False {
          }
          frame True {
            n233 = stacked-sequence {
              tunnel: w335 -> [w342 _]
              tunnel: w334 -> [w341 _]
              tunnel: [w340 _] -> w333
              tunnel: [w339 _] -> w332
              tunnel: [w338 _] -> w331
              frame #0 {
                n234 = call "Show Window.vi"("error in (no error)"=w341, "window refnum (NaWR)"=w342) -> ("error out"=w337:errorcluster, "window refnum out"=w345:T9)  [unwired: 4 in]
                n235 = call "Move Window to Top.vi"("error in (no error)"=w337, "activate? (T)"=TRUE ("activate? (F)"), "window refnum (NaWR)"=w345) -> ("error out"=w336:errorcluster, "window refnum out"=w344:T9)  [unwired: 3 in]
                n236 = call "Get Window Rectangle.vi"("error in (no error)"=w336, "window refnum (NaWR)"=w344) -> ("error out"=w339:errorcluster, "window rect"=w338:T2, "window refnum out"=w340:T9)  [unwired: 3 in]
              }
              frame #1 {
                w346 = u32 1 items=["Down/Press", "Down then Up", "Up/Release"] ("Action")
                n237 = call "Simulate Keyboard.vi"("Action"=w346, "Virtual Key"=u8 65) -> ()  [unwired: 7 in, 1 out]
              }
            }
            n238 = local write "window rect 2"(w331) -> ()
            n239 = call "Show Window.vi"("error in (no error)"=w332, "window refnum (NaWR)"=w333) -> ()  [unwired: 4 in, 2 out]
          }
        }
      }
      event "ZoomIn": Value Change {
        w353 = "WebSDR" ("Such-String")
        n240 = event-data() -> ()  [unwired: 1 in, 6 out]
        n241 = local read "Window title"() -> (w351:string)
        n242 = call "Get Window RefNum.vi"("window name (\"\")"=w351) -> ("error out"=w348:errorcluster, "window refnum (NaWR)"=w349:T9)  [unwired: 7 in]
        n243 = Match Pattern(string=w351, regular expression=w353) -> (match substring=w352:string)  [unwired: 1 in, 3 out]
        n244 = Equal?(x=w352, y=w353) -> (x = y?=w350:bool)
        n245 = case shown="True" w350 {
          tunnel: w349 -> [_ w358]
          tunnel: w348 -> [_ w357]
          frame False {
          }
          frame True {
            n246 = stacked-sequence {
              tunnel: w358 -> [w365 _ _ _]
              tunnel: w357 -> [w364 _ _ _]
              tunnel: [w363 _ _ _] -> w356
              tunnel: [w362 _ _ _] -> w355
              tunnel: [w361 _ _ _] -> w354
              frame #0 {
                n247 = call "Show Window.vi"("error in (no error)"=w364, "window refnum (NaWR)"=w365) -> ("error out"=w360:errorcluster, "window refnum out"=w368:T9)  [unwired: 4 in]
                n248 = call "Move Window to Top.vi"("error in (no error)"=w360, "activate? (T)"=TRUE ("activate? (F)"), "window refnum (NaWR)"=w368) -> ("error out"=w359:errorcluster, "window refnum out"=w367:T9)  [unwired: 3 in]
                n249 = call "Get Window Rectangle.vi"("error in (no error)"=w359, "window refnum (NaWR)"=w367) -> ("error out"=w362:errorcluster, "window rect"=w361:T2, "window refnum out"=w363:T9)  [unwired: 3 in]
              }
              frame #1 {
                w369 = u32 0 items=["Down/Press", "Down then Up", "Up/Release"] ("Action")
                n250 = call "Simulate Keyboard.vi"("Action"=w369, "Virtual Key"=u8 160) -> ()  [unwired: 7 in, 1 out]
              }
              frame #2 {
                w371 = u32 1 items=["Down/Press", "Down then Up", "Up/Release"] ("Action")
                n251 = call "Simulate Keyboard.vi"("Action"=w371, "Virtual Key"=u8 90) -> ()  [unwired: 7 in, 1 out]
              }
              frame #3 {
                w373 = u32 2 items=["Down/Press", "Down then Up", "Up/Release"] ("Action")
                n252 = call "Simulate Keyboard.vi"("Action"=w373, "Virtual Key"=u8 160) -> ()  [unwired: 7 in, 1 out]
              }
            }
            n253 = local write "window rect 2"(w354) -> ()
            n254 = call "Show Window.vi"("error in (no error)"=w355, "window refnum (NaWR)"=w356) -> ()  [unwired: 4 in, 2 out]
          }
        }
      }
      event "ZoomOut": Value Change {
        w380 = "WebSDR" ("Such-String")
        n255 = event-data() -> ()  [unwired: 1 in, 6 out]
        n256 = local read "Window title"() -> (w378:string)
        n257 = call "Get Window RefNum.vi"("window name (\"\")"=w378) -> ("error out"=w375:errorcluster, "window refnum (NaWR)"=w376:T9)  [unwired: 7 in]
        n258 = Match Pattern(string=w378, regular expression=w380) -> (match substring=w379:string)  [unwired: 1 in, 3 out]
        n259 = Equal?(x=w379, y=w380) -> (x = y?=w377:bool)
        n260 = case shown="True" w377 {
          tunnel: w376 -> [_ w385]
          tunnel: w375 -> [_ w384]
          frame False {
          }
          frame True {
            n261 = stacked-sequence {
              tunnel: w385 -> [w392 _]
              tunnel: w384 -> [w391 _]
              tunnel: [w390 _] -> w383
              tunnel: [w389 _] -> w382
              tunnel: [w388 _] -> w381
              frame #0 {
                n262 = call "Show Window.vi"("error in (no error)"=w391, "window refnum (NaWR)"=w392) -> ("error out"=w387:errorcluster, "window refnum out"=w395:T9)  [unwired: 4 in]
                n263 = call "Move Window to Top.vi"("error in (no error)"=w387, "activate? (T)"=TRUE ("activate? (F)"), "window refnum (NaWR)"=w395) -> ("error out"=w386:errorcluster, "window refnum out"=w394:T9)  [unwired: 3 in]
                n264 = call "Get Window Rectangle.vi"("error in (no error)"=w386, "window refnum (NaWR)"=w394) -> ("error out"=w389:errorcluster, "window rect"=w388:T2, "window refnum out"=w390:T9)  [unwired: 3 in]
              }
              frame #1 {
                w396 = u32 1 items=["Down/Press", "Down then Up", "Up/Release"] ("Action")
                n265 = call "Simulate Keyboard.vi"("Action"=w396, "Virtual Key"=u8 90) -> ()  [unwired: 7 in, 1 out]
              }
            }
            n266 = local write "window rect 2"(w381) -> ()
            n267 = call "Show Window.vi"("error in (no error)"=w382, "window refnum (NaWR)"=w383) -> ()  [unwired: 4 in, 2 out]
          }
        }
      }
      event "OpenWebSDR": Value Change {
        n268 = event-data() -> ()  [unwired: 1 in, 6 out]
        n269 = stacked-sequence {
          frame #0 {
            n270 = while {
              stop <- w399 stop-if-true
              n271 = call "You selected a WebSDR- site for your Satellite-operations"() -> ("OK"=w399:bool)  [unwired: 18 in, 1 out]
              n272 = Wait (ms)(milliseconds to wait=u32 500) -> ()  [unwired: 1 out]
            }
          }
          frame #1 {
            (unwired) "C:\\Program Files\\Mozilla Firefox\\firefox.exe "
            n273 = disable-structure shown="Disabled" {
              frame Disabled {
                n274 = call-poly <vilib>:"Open URL in Default Browser.vi"("URL"="http://websdr.is0grb.it:8902/") -> ()  [unwired: 5 in, 2 out]
              }
              frame Enabled {
              }
            }
            n275 = local read "WebSDRDB"() -> (w417:string[][])
            n276 = Transpose 2D Array(2D array=w417) -> (transposed array=w418:string[][])
            n277 = local read "Path of the webbrowser to start WebSDR"() -> (w404:path)
            n278 = Index Array(array=w418, index (row) #1=1 ("index (row)"), index (row) #2=2 ("index (row)"), index (row) #3=3 ("index (row)")) -> (element #1=w408:string[], element #2=w416:string[], element #3=w411:string[])  [unwired: 3 in]
            n279 = property on="WebPages" class="Ring (strict)"() -> ("Value"=w407:u16)  [unwired: 2 in, 2 out]
            n280 = Index Array(array=w408, index=w407) -> (element=w400:string)
            n281 = Index Array(array=w416, index=w407) -> (element=w402:string)
            n282 = Index Array(array=w411, index=w407) -> (element=w410:string)
            n283 = Path To String(path=w404) -> (string=w403:string)
            n284 = Decimal String To Number(string=w410) -> (number=w412:i32)  [unwired: 2 in, 1 out]
            n285 = Concatenate Strings(w403, " " ("string"), w402) -> (w414:string)
            n286 = local write "Truncate Left digits"(w412) -> ()
            n287 = local write "Window title"(w400) -> ()
            n288 = property on="Window title" class="Str"("Value"=w400) -> ()  [unwired: 2 in, 2 out]
            n289 = call <vilib>:"System Exec.vi"("wait until completion? (T)"=FALSE, "command line"=w414) -> ("standard error"=w406:string, "standard output"=w405:string)  [unwired: 6 in, 2 out]
            n290 = local write "standard output"(w405) -> ()
            n291 = local write "standard error"(w406) -> ()
          }
        }
      }
      event "Start browser": Value Change {
        (unwired) "C:\\Program Files\\Mozilla Firefox\\firefox.exe "
        n292 = event-data() -> ()  [unwired: 1 in, 6 out]
        n293 = local read "Path of the webbrowser to start WebSDR"() -> (w424:path)
        n294 = Path To String(path=w424) -> (string=w423:string)
        n295 = Concatenate Strings(w423, " ", "http://websdr.org" ("URL")) -> (w425:string)
        n296 = call <vilib>:"System Exec.vi"("command line"=w425) -> ("standard error"=w427:string, "standard output"=w426:string)  [unwired: 7 in, 2 out]
        n297 = local write "standard output"(w426) -> ()
        n298 = local write "standard error"(w427) -> ()
      }
      event "preferences": Value Change {
        n299 = event-data() -> ()  [unwired: 1 in, 6 out]
        n300 = local write "Tab Control"(T1."Page 2" ("Tab Control")) -> ()
      }
      event "load": Value Change {
        n301 = event-data() -> ()  [unwired: 1 in, 6 out]
        n302 = local write "Tab Control"(T1."Page 3" ("Tab Control")) -> ()
        n303 = call "Current VIs Parent Directory__ogtk.vi"() -> ("Parent Directory (+ Relative)"=w429:path)  [unwired: 5 in]
        n304 = local write "Load controlfile"(w429) -> ()
      }
      event "Load_button": Value Change {
        n305 = event-data() -> ()  [unwired: 1 in, 6 out]
        n306 = stacked-sequence {
          frame #0 {
            n307 = local read "Load controlfile"() -> (w432:path)
            n308 = invoke class="VI" method="Ctrl Val.Get All"(error in=errorcluster {"status"=FALSE, "code"=0, "source"=""} ("error in (no error)"), "Controls"=TRUE) -> (error out=w440:errorcluster, "Get All Control Values Variant"=w437:cluster{"Name":string, "Variant Data":variant}[])  [unwired: 2 in, 2 out]
            n309 = call <vilib>:"Read Characters From File.vi"("file path (dialog if empty)"=w432) -> ("character string"=w433:string)  [unwired: 5 in, 3 out]
            n310 = Unflatten From String(type=w437, binary string=w433, data includes array or string size? (T)=TRUE, error in (no error)=w440) -> (value=w435:cluster{"Name":string, "Variant Data":variant}[], error out=w438:errorcluster)  [unwired: 1 in, 1 out]
            n311 = for {
              tunnel: w435 -> [w445] mode=indexing
              tunnel: w438 -> [w442]
              tunnel: [w441] -> w439
              n312 = Unbundle By Name(w445) -> ("Name"=w443:string, "Variant Data"=w444:variant)
              n313 = invoke class="VI" method="Ctrl Val.Set"(error in=w442, "Control Name"=w443, "Value"=w444) -> (error out=w441:errorcluster)  [unwired: 2 in, 4 out]
            }
            "error out 3" <- w439
          }
          frame #1 {
            n314 = local write "Tab Control"(T1."Page 1" ("Tab Control")) -> ()
          }
        }
      }
      event "goback_button": Value Change {
        n315 = event-data() -> ()  [unwired: 1 in, 6 out]
        n316 = stacked-sequence {
          frame #0 {
            w452 = "websdr" ("regular expression")
            n317 = property class="VI"() -> ("VI-Name"=w462:string)  [unwired: 2 in, 2 out]
            n318 = call "Current VIs Parent Directory__ogtk.vi"() -> ("Parent Directory (+ Relative)"=w474:path)  [unwired: 5 in]
            n319 = String Length(string=w462) -> (length=w460:i32)
            n320 = Subtract(x=w460, y=3) -> (x-y=w461:i32)
            n321 = String Subset(string=w462, length (rest)=w461) -> (substring=w481:string)  [unwired: 1 in]
            n322 = Concatenate Strings(w481, "*" ("string")) -> (w479:string)
            n323 = List Folder(path=w474, pattern=w479) -> (filenames=w480:string[])  [unwired: 2 in, 3 out]
            n324 = for {
              tunnel: w480 -> [w482] mode=indexing
              tunnel: w452 -> [w485]
              tunnel: [w484] -> w468 mode=indexing
              tunnel: [w482] -> _ mode=indexing
              n325 = Match Pattern(string=w482, regular expression=w485) -> (after substring=w483:string)  [unwired: 1 in, 3 out]
              n326 = Decimal String To Number(string=w483) -> (number=w484:i32)  [unwired: 2 in, 1 out]
            }
            n327 = Concatenate Strings(w481, ".ctr" ("String")) -> (w478:string)
            n328 = Build Path(base path=w474, name or relative path=w478) -> (appended path=w456:path)
            n329 = Array Max & Min(array=w468) -> (max value=w477:i32)  [unwired: 3 out]
            n330 = Concatenate Strings(w462, "\\" ("string")) -> (w459:string)
            n331 = Path To String(path=w456) -> (string=w457:string)
            n332 = Increment(x=w477) -> (x+1=w467:i32)
            n333 = Search and Replace String(input string=w457, search string=w459) -> (result string=w458:string)  [unwired: 6 in, 3 out]
            n334 = Format Value(format string="%03d", value (0)=w467) -> (output string=w466:string)  [unwired: 1 in]
            n335 = String To Path(string=w458) -> (path=w463:path)
            "path 3" <- w463
            n336 = local write "path"(w463) -> ()
            n337 = Concatenate Strings(w452, w466) -> (w476:string)
            n338 = Concatenate Strings(w476, ".ctr" ("String")) -> (w469:string)
            n339 = invoke class="VI" method="Ctrl Val.Get All"("Controls"=TRUE ("controls")) -> ("Get All Control Values Variant"=w464:cluster{"Name":string, "Variant Data":variant}[])  [unwired: 3 in, 3 out]
            n340 = Build Path(base path=w474, name or relative path=w469) -> (appended path=w473:path)
            n341 = Concatenate Strings(w476, "\\" ("string")) -> (w470:string)
            n342 = Path To String(path=w473) -> (string=w472:string)
            n343 = Search and Replace String(input string=w472, search string=w470) -> (result string=w471:string)  [unwired: 6 in, 3 out]
            n344 = Flatten To String(anything=w464) -> (data string=w465:string)  [unwired: 3 in, 2 out]
            n345 = String To Path(string=w471) -> (path=w475:path)
            n346 = stacked-sequence {
              tunnel: w463 -> [_ w490 _ w493 _]
              tunnel: w465 -> [w486 _ _ w492 _]
              tunnel: w475 -> [w487 _ _ _ _]
              frame #0 {
                n347 = call <vilib>:"Write Characters To File.vi"("character string"=w486, "file path (dialog if empty)"=w487) -> ()  [unwired: 3 in, 1 out]
              }
              frame #1 {
                w489 = T5 0 items=["no dialog", "OK message", "continue or stop message", "OK message + warnings", "continue/stop + warnings"] ("type of dialog (OK msg:1)")
                n348 = Delete(path (use dialog)=w490) -> (error out=w488:errorcluster)  [unwired: 4 in, 2 out]
                n349 = call <vilib>:"Simple Error Handler.vi"("type of dialog (OK msg:1)"=w489, "error in (no error)"=w488) -> ()  [unwired: 3 in, 5 out]
              }
              frame #2 {
                n350 = Wait (ms)(milliseconds to wait=u32 2000) -> ()  [unwired: 1 out]
              }
              frame #3 {
                n351 = call <vilib>:"Write Characters To File.vi"("character string"=w492, "file path (dialog if empty)"=w493) -> ()  [unwired: 3 in, 1 out]
              }
              frame #4 {
                n352 = Wait (ms)(milliseconds to wait=u32 2000) -> ()  [unwired: 1 out]
              }
            }
          }
          frame #1 {
            n353 = local write "Tab Control"(T1."Page 1" ("Tab Control")) -> ()
          }
          frame #2 {
            n354 = One Button Dialog(message="Orbitron2WebSDR will be stoped \nand must be restarted", button name ("OK")="Copy") -> (true=w496:bool)
            n355 = Stop(stop? (T)=w496) -> ()
          }
        }
      }
      event "FocusWebSDR": Value Change {
        n356 = event-data() -> ()  [unwired: 1 in, 6 out]
        n357 = flat-sequence {
          frame #0 {
            n358 = property on="processes Box" class="CmbBox"() -> ("Text.Text"=w504:string)  [unwired: 2 in, 2 out]
            n359 = local write "Window title"(w504) -> ()
            n360 = call "Get Window RefNum.vi"("window name (\"\")"=w504) -> ("error out"=w500:errorcluster, "window refnum (NaWR)"=w501:T9)  [unwired: 7 in]
            n361 = call "Show Window.vi"("error in (no error)"=w500, "window refnum (NaWR)"=w501) -> ("error out"=w503:errorcluster, "window refnum out"=w502:T9)  [unwired: 4 in]
            n362 = call "Move Window to Top.vi"("error in (no error)"=w503, "activate? (T)"=TRUE ("activate? (F)"), "window refnum (NaWR)"=w502) -> ()  [unwired: 3 in, 2 out]
          }
          frame #1 {
            n363 = call "You selected a WebSDR- site for your Satellite-operations2"() -> ()  [unwired: 18 in, 2 out]
          }
        }
      }
      event "AddWebSDR": Value Change {
        w507 = ""
        w510 = FALSE
        w509 = TRUE
        n364 = event-data() -> ()  [unwired: 1 in, 6 out]
        n365 = local read "Truncate Left digits"() -> (w512:i32)
        n366 = local read "Downlink corr."() -> (w506:dbl)
        n367 = local write "WebSDR Location / Name"(w507) -> ()
        n368 = local write "Tab Control"(enum32{"Page 1", "Page 2", "Page 3", "Page 4"}."Page 4" ("Tab Control")) -> ()
        n369 = Number To Fractional String(number=w506) -> (F-format string=w505:string)  [unwired: 3 in]
        n370 = local write "WebSDR URL"(w507) -> ()
        n371 = Number To Decimal String(number=w512) -> (decimal integer string=w511:string)  [unwired: 1 in]
        n372 = local write "Downlink corr."(w505) -> ()
        n373 = local write "Truncate digits"(w511) -> ()
        n374 = local write "Title"("Add a new WebSDR database item" ("Title")) -> ()
        n375 = property on="Cancel Add" class="Bool"("Visible"=w509) -> ()  [unwired: 2 in, 2 out]
        n376 = property on="Add_Button" class="Bool"("Visible"=w509) -> ()  [unwired: 2 in, 2 out]
        n377 = property on="Cancel Edit" class="Bool"("Visible"=w510) -> ()  [unwired: 2 in, 2 out]
        n378 = property on="Edit_Button" class="Bool"("Visible"=w510) -> ()  [unwired: 2 in, 2 out]
      }
      event "Add_Button": Value Change {
        n379 = event-data() -> ()  [unwired: 1 in, 6 out]
        n380 = stacked-sequence {
          frame #0 {
            n381 = local read "WebSDR Location / Name"() -> (w519:string)
            n382 = local read "WebSDRDB"() -> (w523:string[][])
            n383 = local read "WebSDR URL"() -> (w515:string)
            n384 = local read "Window title"() -> (w522:string)
            n385 = local read "Downlink corr."() -> (w514:string)
            n386 = local read "Truncate digits"() -> (w520:string)
            n387 = Build Array(w519, w522, w515, w520, w514) -> (w521:string[])
            n388 = Insert Into Array(array=w523, new element=w521) -> (w517:string[][])  [unwired: 2 in]
            n389 = local write "WebSDRDB"(w517) -> ()
            n390 = Transpose 2D Array(2D array=w517) -> (transposed array=w516:string[][])
            n391 = Index Array(array=w516) -> (element=w518:string[])  [unwired: 2 in]
            n392 = property on="WebPages" class="Ring (strict)"("Strings []"=w518) -> ()  [unwired: 2 in, 2 out]
          }
          frame #1 {
            n393 = local write "Tab Control"(enum32{"Page 1", "Page 2", "Page 3", "Page 4"}."Page 1" ("Tab Control")) -> ()
            n394 = property on="WebPages" class="Ring (strict)"("Value"=0) -> ()  [unwired: 2 in, 2 out]
          }
          frame #2 {
            w542 = "websdrOrbitron" ("regular expression")
            n395 = property class="VI"() -> ("VI-Name"=w537:string)  [unwired: 2 in, 2 out]
            n396 = String Length(string=w537) -> (length=w532:i32)
            n397 = call "Current VIs Parent Directory__ogtk.vi"() -> ("Parent Directory (+ Relative)"=w557:path)  [unwired: 5 in]
            n398 = Subtract(x=w532, y=3) -> (x-y=w534:i32)
            n399 = String Subset(string=w537, length (rest)=w534) -> (substring=w547:string)  [unwired: 1 in]
            n400 = Concatenate Strings(w547, "*" ("string")) -> (w549:string)
            n401 = List Folder(path=w557, pattern=w549) -> (filenames=w526:string[])  [unwired: 2 in, 3 out]
            n402 = for {
              tunnel: w526 -> [w564] mode=indexing
              tunnel: w542 -> [w563]
              tunnel: [w561] -> w546 mode=indexing
              n403 = Match Pattern(string=w564, regular expression=w563) -> (after substring=w562:string)  [unwired: 1 in, 3 out]
              n404 = Decimal String To Number(string=w562) -> (number=w561:i32)  [unwired: 2 in, 1 out]
            }
            n405 = Concatenate Strings(w547, ".ctr" ("String")) -> (w536:string)
            n406 = Build Path(base path=w557, name or relative path=w536) -> (appended path=w527:path)
            n407 = Concatenate Strings(w537, "\\" ("string")) -> (w531:string)
            n408 = Array Max & Min(array=w546) -> (max value=w560:i32)  [unwired: 3 out]
            n409 = Path To String(path=w527) -> (string=w528:string)
            n410 = Increment(x=w560) -> (x+1=w545:i32)
            n411 = Search and Replace String(input string=w528, search string=w531) -> (result string=w529:string)  [unwired: 6 in, 3 out]
            n412 = String To Path(string=w529) -> (path=w538:path)
            n413 = Format Value(format string="%03d", value (0)=w545) -> (output string=w543:string)  [unwired: 1 in]
            n414 = local write "path"(w538) -> ()
            n415 = Concatenate Strings(w542, w543) -> (w559:string)
            n416 = Concatenate Strings(w559, ".ctr" ("String")) -> (w550:string)
            n417 = Build Path(base path=w557, name or relative path=w550) -> (appended path=w556:path)
            n418 = Concatenate Strings(w559, "\\" ("string")) -> (w552:string)
            n419 = invoke class="VI" method="Ctrl Val.Get All"("Controls"=TRUE ("controls")) -> ("Get All Control Values Variant"=w539:cluster{"Name":string, "Variant Data":variant}[])  [unwired: 3 in, 3 out]
            n420 = Path To String(path=w556) -> (string=w555:string)
            n421 = Search and Replace String(input string=w555, search string=w552) -> (result string=w554:string)  [unwired: 6 in, 3 out]
            n422 = String To Path(string=w554) -> (path=w558:path)
            n423 = Flatten To String(anything=w539) -> (data string=w541:string)  [unwired: 3 in, 2 out]
            n424 = stacked-sequence {
              tunnel: w538 -> [_ w569 w571]
              tunnel: w541 -> [w565 _ w570]
              tunnel: w558 -> [w566 _ _]
              frame #0 {
                n425 = call <vilib>:"Write Characters To File.vi"("character string"=w565, "file path (dialog if empty)"=w566) -> ()  [unwired: 3 in, 1 out]
              }
              frame #1 {
                w568 = T5 0 items=["no dialog", "OK message", "continue or stop message", "OK message + warnings", "continue/stop + warnings"] ("type of dialog (OK msg:1)")
                n426 = Delete(path (use dialog)=w569) -> (error out=w567:errorcluster)  [unwired: 4 in, 2 out]
                n427 = call <vilib>:"Simple Error Handler.vi"("type of dialog (OK msg:1)"=w568, "error in (no error)"=w567) -> ()  [unwired: 3 in, 5 out]
              }
              frame #2 {
                n428 = call <vilib>:"Write Characters To File.vi"("character string"=w570, "file path (dialog if empty)"=w571) -> ()  [unwired: 3 in, 1 out]
              }
            }
          }
        }
      }
      event "Edit_Button": Value Change {
        n429 = event-data() -> ()  [unwired: 1 in, 6 out]
        n430 = stacked-sequence {
          frame #0 {
            n431 = local read "WebSDR Location / Name"() -> (w579:string)
            n432 = local read "WebSDRDB"() -> (w582:string[][])
            n433 = local read "WebSDR URL"() -> (w575:string)
            n434 = local read "Window title"() -> (w581:string)
            n435 = local read "Downlink corr."() -> (w572:string)
            n436 = local read "Truncate digits"() -> (w580:string)
            n437 = property on="WebPages" class="Ring (strict)"() -> ("Value"=w574:u16)  [unwired: 2 in, 2 out]
            n438 = Build Array(w579, w581, w575, w580, w572) -> (w573:string[])
            n439 = Replace Array Subset(array=w582, new element=w573, index (row)=w574) -> (w577:string[][])  [unwired: 1 in]
            n440 = Transpose 2D Array(2D array=w577) -> (transposed array=w576:string[][])
            n441 = local write "WebSDRDB"(w577) -> ()
            n442 = Index Array(array=w576) -> (element=w578:string[])  [unwired: 2 in]
            n443 = property on="WebPages" class="Ring (strict)"("Strings []"=w578) -> ()  [unwired: 2 in, 2 out]
          }
          frame #1 {
            n444 = local write "Tab Control"(enum32{"Page 1", "Page 2", "Page 3", "Page 4"}."Page 1" ("Tab Control")) -> ()
            n445 = property on="WebPages" class="Ring (strict)"("Value"=0) -> ()  [unwired: 2 in, 2 out]
          }
          frame #2 {
            w601 = "websdrOrbitron" ("regular expression")
            n446 = property class="VI"() -> ("VI-Name"=w596:string)  [unwired: 2 in, 2 out]
            n447 = String Length(string=w596) -> (length=w591:i32)
            n448 = call "Current VIs Parent Directory__ogtk.vi"() -> ("Parent Directory (+ Relative)"=w616:path)  [unwired: 5 in]
            n449 = Subtract(x=w591, y=3) -> (x-y=w593:i32)
            n450 = String Subset(string=w596, length (rest)=w593) -> (substring=w606:string)  [unwired: 1 in]
            n451 = Concatenate Strings(w606, "*" ("string")) -> (w608:string)
            n452 = List Folder(path=w616, pattern=w608) -> (filenames=w585:string[])  [unwired: 2 in, 3 out]
            n453 = for {
              tunnel: w585 -> [w623] mode=indexing
              tunnel: w601 -> [w622]
              tunnel: [w620] -> w605 mode=indexing
              n454 = Match Pattern(string=w623, regular expression=w622) -> (after substring=w621:string)  [unwired: 1 in, 3 out]
              n455 = Decimal String To Number(string=w621) -> (number=w620:i32)  [unwired: 2 in, 1 out]
            }
            n456 = Concatenate Strings(w606, ".ctr" ("String")) -> (w595:string)
            n457 = Build Path(base path=w616, name or relative path=w595) -> (appended path=w586:path)
            n458 = Concatenate Strings(w596, "\\" ("string")) -> (w590:string)
            n459 = Array Max & Min(array=w605) -> (max value=w619:i32)  [unwired: 3 out]
            n460 = Path To String(path=w586) -> (string=w587:string)
            n461 = Increment(x=w619) -> (x+1=w604:i32)
            n462 = Search and Replace String(input string=w587, search string=w590) -> (result string=w588:string)  [unwired: 6 in, 3 out]
            n463 = String To Path(string=w588) -> (path=w597:path)
            n464 = Format Value(format string="%03d", value (0)=w604) -> (output string=w602:string)  [unwired: 1 in]
            n465 = local write "path"(w597) -> ()
            n466 = Concatenate Strings(w601, w602) -> (w618:string)
            n467 = Concatenate Strings(w618, ".ctr" ("String")) -> (w609:string)
            n468 = Build Path(base path=w616, name or relative path=w609) -> (appended path=w615:path)
            n469 = Concatenate Strings(w618, "\\" ("string")) -> (w611:string)
            n470 = invoke class="VI" method="Ctrl Val.Get All"("Controls"=TRUE ("controls")) -> ("Get All Control Values Variant"=w598:cluster{"Name":string, "Variant Data":variant}[])  [unwired: 3 in, 3 out]
            n471 = Path To String(path=w615) -> (string=w614:string)
            n472 = Search and Replace String(input string=w614, search string=w611) -> (result string=w613:string)  [unwired: 6 in, 3 out]
            n473 = String To Path(string=w613) -> (path=w617:path)
            n474 = Flatten To String(anything=w598) -> (data string=w600:string)  [unwired: 3 in, 2 out]
            n475 = stacked-sequence {
              tunnel: w597 -> [_ w628 w630]
              tunnel: w600 -> [w624 _ w629]
              tunnel: w617 -> [w625 _ _]
              frame #0 {
                n476 = call <vilib>:"Write Characters To File.vi"("character string"=w624, "file path (dialog if empty)"=w625) -> ()  [unwired: 3 in, 1 out]
              }
              frame #1 {
                w627 = T5 0 items=["no dialog", "OK message", "continue or stop message", "OK message + warnings", "continue/stop + warnings"] ("type of dialog (OK msg:1)")
                n477 = Delete(path (use dialog)=w628) -> (error out=w626:errorcluster)  [unwired: 4 in, 2 out]
                n478 = call <vilib>:"Simple Error Handler.vi"("type of dialog (OK msg:1)"=w627, "error in (no error)"=w626) -> ()  [unwired: 3 in, 5 out]
              }
              frame #2 {
                n479 = call <vilib>:"Write Characters To File.vi"("character string"=w629, "file path (dialog if empty)"=w630) -> ()  [unwired: 3 in, 1 out]
              }
            }
          }
        }
      }
      event "DeleteWebSDR": Value Change {
        n480 = event-data() -> ()  [unwired: 1 in, 6 out]
        n481 = property on="WebPages" class="Ring (strict)"() -> ("RingText.Text"=w632:string)  [unwired: 2 in, 2 out]
        n482 = Concatenate Strings("Are you sure to delete the Mode specification:\n" ("message"), w632, "?" ("string")) -> (w637:string)
        n483 = Two Button Dialog(message=w637, 1:"No" ("F button name (\"Cancel\")"), 2:"Yes" ("T button name (\"OK\")")) -> (T button?=w631:bool)
        n484 = case shown="True" w631 {
          frame False {
          }
          frame True {
            n485 = stacked-sequence {
              frame #0 {
                n486 = local read "WebSDRDB"() -> (w640:string[][])
                n487 = property on="WebPages" class="Ring (strict)"() -> ("Value"=w638:u16)  [unwired: 2 in, 2 out]
                n488 = Delete From Array(array=w640, index (row)=w638) -> (array with subset deleted=w639:string[][])  [unwired: 2 in, 1 out]
                n489 = local write "WebSDRDB"(w639) -> ()
              }
              frame #1 {
                n490 = property on="WebPages" class="Ring (strict)"("Value"=0) -> ()  [unwired: 2 in, 2 out]
                n491 = local write "Tab Control"(enum32{"Page 1", "Page 2", "Page 3", "Page 4"}."Page 1" ("Tab Control")) -> ()
              }
              frame #2 {
                w659 = "websdrOrbitron" ("regular expression")
                n492 = property class="VI"() -> ("VI-Name"=w654:string)  [unwired: 2 in, 2 out]
                n493 = String Length(string=w654) -> (length=w649:i32)
                n494 = call "Current VIs Parent Directory__ogtk.vi"() -> ("Parent Directory (+ Relative)"=w674:path)  [unwired: 5 in]
                n495 = Subtract(x=w649, y=3) -> (x-y=w651:i32)
                n496 = String Subset(string=w654, length (rest)=w651) -> (substring=w664:string)  [unwired: 1 in]
                n497 = Concatenate Strings(w664, "*" ("string")) -> (w666:string)
                n498 = List Folder(path=w674, pattern=w666) -> (filenames=w643:string[])  [unwired: 2 in, 3 out]
                n499 = for {
                  tunnel: w643 -> [w681] mode=indexing
                  tunnel: w659 -> [w680]
                  tunnel: [w678] -> w663 mode=indexing
                  n500 = Match Pattern(string=w681, regular expression=w680) -> (after substring=w679:string)  [unwired: 1 in, 3 out]
                  n501 = Decimal String To Number(string=w679) -> (number=w678:i32)  [unwired: 2 in, 1 out]
                }
                n502 = Concatenate Strings(w664, ".ctr" ("String")) -> (w653:string)
                n503 = Build Path(base path=w674, name or relative path=w653) -> (appended path=w644:path)
                n504 = Concatenate Strings(w654, "\\" ("string")) -> (w648:string)
                n505 = Array Max & Min(array=w663) -> (max value=w677:i32)  [unwired: 3 out]
                n506 = Path To String(path=w644) -> (string=w645:string)
                n507 = Increment(x=w677) -> (x+1=w662:i32)
                n508 = Search and Replace String(input string=w645, search string=w648) -> (result string=w646:string)  [unwired: 6 in, 3 out]
                n509 = String To Path(string=w646) -> (path=w655:path)
                n510 = Format Value(format string="%03d", value (0)=w662) -> (output string=w660:string)  [unwired: 1 in]
                n511 = local write "path"(w655) -> ()
                n512 = Concatenate Strings(w659, w660) -> (w676:string)
                n513 = Concatenate Strings(w676, ".ctr" ("String")) -> (w667:string)
                n514 = Build Path(base path=w674, name or relative path=w667) -> (appended path=w673:path)
                n515 = Concatenate Strings(w676, "\\" ("string")) -> (w669:string)
                n516 = invoke class="VI" method="Ctrl Val.Get All"("Controls"=TRUE ("controls")) -> ("Get All Control Values Variant"=w656:cluster{"Name":string, "Variant Data":variant}[])  [unwired: 3 in, 3 out]
                n517 = Path To String(path=w673) -> (string=w672:string)
                n518 = Search and Replace String(input string=w672, search string=w669) -> (result string=w671:string)  [unwired: 6 in, 3 out]
                n519 = String To Path(string=w671) -> (path=w675:path)
                n520 = Flatten To String(anything=w656) -> (data string=w658:string)  [unwired: 3 in, 2 out]
                n521 = stacked-sequence {
                  tunnel: w655 -> [_ w686 w688]
                  tunnel: w658 -> [w682 _ w687]
                  tunnel: w675 -> [w683 _ _]
                  frame #0 {
                    n522 = call <vilib>:"Write Characters To File.vi"("character string"=w682, "file path (dialog if empty)"=w683) -> ()  [unwired: 3 in, 1 out]
                  }
                  frame #1 {
                    w685 = T5 0 items=["no dialog", "OK message", "continue or stop message", "OK message + warnings", "continue/stop + warnings"] ("type of dialog (OK msg:1)")
                    n523 = Delete(path (use dialog)=w686) -> (error out=w684:errorcluster)  [unwired: 4 in, 2 out]
                    n524 = call <vilib>:"Simple Error Handler.vi"("type of dialog (OK msg:1)"=w685, "error in (no error)"=w684) -> ()  [unwired: 3 in, 5 out]
                  }
                  frame #2 {
                    n525 = call <vilib>:"Write Characters To File.vi"("character string"=w687, "file path (dialog if empty)"=w688) -> ()  [unwired: 3 in, 1 out]
                  }
                }
              }
            }
          }
        }
      }
      event "Cancel load", "Cancel Edit", "Cancel Edit 2": Value Change {
        n526 = event-data() -> ()  [unwired: 1 in, 6 out]
        n527 = local write "Tab Control"(enum32{"Page 1", "Page 2", "Page 3", "Page 4"}."Page 1" ("Tab Control")) -> ()
      }
      event "EditWebSDR": Value Change {
        w690 = TRUE
        w692 = FALSE
        n528 = event-data() -> ()  [unwired: 1 in, 6 out]
        n529 = local read "WebSDRDB"() -> (w706:string[][])
        n530 = Transpose 2D Array(2D array=w706) -> (transposed array=w707:string[][])
        n531 = local write "Tab Control"(enum32{"Page 1", "Page 2", "Page 3", "Page 4"}."Page 4" ("Tab Control")) -> ()
        n532 = Index Array(array=w707, index (row) #1=0 ("index (row)"), index (row) #2=1 ("index (row)"), index (row) #3=2 ("index (row)"), index (row) #4=3 ("index (row)")) -> (element #1=w697:string[], element #2=w703:string[], element #3=w705:string[], element #4=w704:string[])  [unwired: 4 in]
        n533 = local write "Title"("Edit WebSDR database item" ("Title")) -> ()
        n534 = property on="WebPages" class="Ring (strict)"() -> ("Value"=w698:u16)  [unwired: 2 in, 2 out]
        n535 = Index Array(array=w697, index=w698) -> (element=w696:string)
        n536 = Index Array(array=w703, index=w698) -> (element=w695:string)
        n537 = Index Array(array=w705, index=w698) -> (element=w694:string)
        n538 = Index Array(array=w704, index=w698) -> (element=w693:string)
        n539 = local write "WebSDR Location / Name"(w696) -> ()
        n540 = local write "Window title"(w695) -> ()
        n541 = local write "WebSDR URL"(w694) -> ()
        n542 = local write "Truncate digits"(w693) -> ()
        n543 = property on="Cancel Add" class="Bool"("Visible"=w692) -> ()  [unwired: 2 in, 2 out]
        n544 = property on="Add_Button" class="Bool"("Visible"=w692) -> ()  [unwired: 2 in, 2 out]
        n545 = property on="Cancel Edit" class="Bool"("Visible"=w690) -> ()  [unwired: 2 in, 2 out]
        n546 = property on="Edit_Button" class="Bool"("Visible"=w690) -> ()  [unwired: 2 in, 2 out]
      }
      event "Stop Cat Control": Value Change {
        w709 = ""
        w711 = TRUE
        w712 = T6."Disabled and Grayed Out" ("Disabled")
        n547 = event-data() -> ()  [unwired: 1 in, 6 out]
        n548 = local write "dont write"(FALSE ("dont write")) -> ()
        n549 = property on="Radio Mode" class="Bool (strict)"("Value"=w711) -> ()  [unwired: 2 in, 2 out]
        n550 = local write "Radio Mode"(w711) -> ()
        n551 = property on="Cat Control" class="Bool (strict)"("DisabledEnum"=T6."Enabled" ("Disabled"), "Value"=FALSE ("Cat Control")) -> ()  [unwired: 2 in, 2 out]
        n552 = property on="ManualLatch" class="Bool"("DisabledEnum"=w712) -> ()  [unwired: 2 in, 2 out]
        n553 = property on="Truncate Left digits" class="DigNum (strict)"("DisabledEnum"=w712) -> ()  [unwired: 2 in, 2 out]
        n554 = property on="Downlink Freq. Man." class="DigNum (strict)"("DisabledEnum"=w712) -> ()  [unwired: 2 in, 2 out]
        n555 = property on="Downlink corr." class="Knob (strict)"("DisabledEnum"=w712) -> ()  [unwired: 2 in, 2 out]
        n556 = property on="Radio Mode" class="Bool (strict)"("DisabledEnum"=w712) -> ()  [unwired: 2 in, 2 out]
        n557 = property on="Downlink Freq." class="Str"("DisabledEnum"=w712) -> ()  [unwired: 2 in, 2 out]
        n558 = property on="Stop Cat Control" class="Bool"("DisabledEnum"=T6."Disabled and Grayed Out" ("Disabled")) -> ()  [unwired: 2 in, 2 out]
        n559 = local write "data"(w709) -> ()
        n560 = property on="data" class="Str"("Value"=w709) -> ()  [unwired: 2 in, 2 out]
        n561 = flat-sequence {
          frame #0 {
            w716 = "Tracking disengaged" ("Lisa")
            n562 = local write "Lisa"(w716) -> ()
            n563 = property on="Lisa" class="Str"("Value"=w716) -> ()  [unwired: 2 in, 2 out]
          }
          frame #1 {
            n564 = Wait (ms)(milliseconds to wait=u32 500) -> ()  [unwired: 1 out]
          }
        }
      }
    }
    n565 = Wait (ms)(milliseconds to wait=u32 250) -> ()  [unwired: 1 out]
  }
  n566 = call-poly <vilib>:"Close Input Device.vi"("error in (no error)"=w2, "device ID"=w3) -> ()  [unwired: 8 in, 1 out]
  n567 = while {
    stop <- w719 stop-if-true
    n568 = control-ref of="Lisa"() -> (w718:refnum<vi>)
    n569 = property on="kill" class="Bool (strict)"() -> ("Value"=w719:bool)  [unwired: 2 in, 2 out]
    n570 = control-ref of="TTS Voice"() -> (w727:refnum<vi>)
    n571 = control-ref of="Output Device"() -> (w726:refnum<vi>)
    n572 = call "Blink when valuechange subvi.vi"("Indicator or ctrl to look up value change"=w718) -> ()  [unwired: 9 in, 2 out]
    n573 = call "TTS_MCC.vi"("Volume"="Volume 2", "Rate"="Rate 2", "Output Device"="Output Device", "reference (Eingang)"=w727, "Lisa"="Lisa", "TTS Voice"="TTS Voice", "Ring (Eingang)"=w726) -> ()  [unwired: 4 in, 1 out]
    n574 = Wait (ms)(milliseconds to wait=u32 500) -> ()  [unwired: 1 out]
  }
  n575 = stacked-sequence {
    tunnel: FALSE ("iterCompleted") -> [_ w745 _ _ _]
    frame #0 {
      n576 = flat-sequence {
        frame #0 {
          n577 = Wait (ms)(milliseconds to wait=u32 1000) -> ()  [unwired: 1 out]
        }
        frame #1 {
          w729 = "Welcome to Orbitron to WebSDR"
          n578 = local write "Lisa"(w729) -> ()
          n579 = property on="Lisa" class="Str"("Value"=w729) -> ()  [unwired: 2 in, 2 out]
        }
        frame #2 {
        }
      }
    }
    frame #1 {
      w732 = T5 0 items=["no dialog", "OK message", "continue or stop message", "OK message + warnings", "continue/stop + warnings"] ("type of dialog (OK msg:1)")
      n580 = property class="VI"(error in=errorcluster {"status"=FALSE, "code"=0, "source"=""} ("error in (no error)")) -> (error out=w735:errorcluster, "VI-Name"=w753:string)  [unwired: 1 in, 1 out]
      n581 = String Length(string=w753) -> (length=w751:i32)
      n582 = local write "iterCompleted"(w745) -> ()
      n583 = local write "slave1Killed"(w745) -> ()
      n584 = local write "slave3Killed"(w745) -> ()
      n585 = local write "slave4Killed"(w745) -> ()
      n586 = Subtract(x=w751, y=3) -> (x-y=w749:i32)
      n587 = String Subset(string=w753, length (rest)=w749) -> (substring=w746:string)  [unwired: 1 in]
      n588 = Concatenate Strings(w746, ".ctr" ("String")) -> (w747:string)
      n589 = call <vilib>:"Application Directory.vi"() -> ("Application Directory"=w733:path)
      n590 = Concatenate Strings(w746, "\\" ("string")) -> (w743:string)
      "concatenated string" <- w743
      n591 = Build Path(base path=w733, name or relative path=w747) -> (appended path=w744:path)
      n592 = Path To String(path=w744) -> (string=w742:string)
      "string" <- w742
      n593 = Search and Replace String(input string=w742, search string=w743) -> (result string=w741:string)  [unwired: 6 in, 3 out]
      n594 = String To Path(string=w741) -> (path=w740:path)
      n595 = call "Current VIs Parent Directory__ogtk.vi"() -> ("Parent Directory (+ Relative)"=w730:path)  [unwired: 5 in]
      n596 = invoke class="VI" method="Ctrl Val.Get All"(error in=w735, "Controls"=TRUE) -> (error out=w734:errorcluster, "Get All Control Values Variant"=w738:cluster{"Name":string, "Variant Data":variant}[])  [unwired: 2 in, 2 out]
      n597 = local write "path 4"(w740) -> ()
      n598 = local write "Parent Directory (+ Relative)"(w730) -> ()
      n599 = call <vilib>:"Read Characters From File.vi"("file path (dialog if empty)"=w740) -> ("character string"=w756:string)  [unwired: 5 in, 3 out]
      n600 = Unflatten From String(type=w738, binary string=w756, data includes array or string size? (T)=TRUE, error in (no error)=w734) -> (value=w754:cluster{"Name":string, "Variant Data":variant}[], error out=w737:errorcluster)  [unwired: 1 in, 1 out]
      n601 = for {
        tunnel: w754 -> [w761] mode=indexing
        tunnel: w737 -> [w758]
        tunnel: [w757] -> w731
        n602 = Unbundle By Name(w761) -> ("Name"=w759:string, "Variant Data"=w760:variant)
        n603 = invoke class="VI" method="Ctrl Val.Set"(error in=w758, "Control Name"=w759, "Value"=w760) -> (error out=w757:errorcluster)  [unwired: 2 in, 4 out]
      }
      "error out 2" <- w731
      n604 = call <vilib>:"Simple Error Handler.vi"("type of dialog (OK msg:1)"=w732, "error in (no error)"=w731) -> ()  [unwired: 3 in, 5 out]
    }
    frame #2 {
      w762 = FALSE
      w766 = ""
      w767 = FALSE ("kill")
      w763 = T6."Disabled and Grayed Out" ("Disabled")
      n605 = local write "Cat Control"(w762) -> ()
      n606 = property on="Cat Control" class="Bool (strict)"("Value"=w762) -> ()  [unwired: 2 in, 2 out]
      n607 = local write "Tab Control"(enum32{"Page 1", "Page 2", "Page 3", "Page 4"}."Page 1" ("Tab Control")) -> ()
      n608 = local write "Satellite Name"(w766) -> ()
      n609 = local write "Radio Mode"(TRUE ("Radio Mode")) -> ()
      n610 = local write "Type of DN"(w766) -> ()
      n611 = local write "dont write"(FALSE ("dont write")) -> ()
      n612 = local write "kill"(w767) -> ()
      n613 = property on="kill" class="Bool (strict)"("Value"=w767) -> ()  [unwired: 2 in, 2 out]
      n614 = local read "WebSDRDB"() -> (w771:string[][])
      n615 = Transpose 2D Array(2D array=w771) -> (transposed array=w772:string[][])
      n616 = Index Array(array=w772) -> (element=w773:string[])  [unwired: 2 in]
      n617 = property on="Cat Control" class="Bool (strict)"("DisabledEnum"=T6."Enabled" ("Disabled"), "Value"=FALSE ("Cat Control")) -> ()  [unwired: 2 in, 2 out]
      n618 = property on="ManualLatch" class="Bool"("DisabledEnum"=w763) -> ()  [unwired: 2 in, 2 out]
      n619 = property on="Truncate Left digits" class="DigNum (strict)"("DisabledEnum"=w763) -> ()  [unwired: 2 in, 2 out]
      n620 = property on="Downlink Freq. Man." class="DigNum (strict)"("DisabledEnum"=w763) -> ()  [unwired: 2 in, 2 out]
      n621 = property on="Downlink corr." class="Knob (strict)"("DisabledEnum"=w763) -> ()  [unwired: 2 in, 2 out]
      n622 = property on="Radio Mode" class="Bool (strict)"("DisabledEnum"=w763) -> ()  [unwired: 2 in, 2 out]
      n623 = property on="Downlink Freq." class="Str"("DisabledEnum"=w763) -> ()  [unwired: 2 in, 2 out]
      n624 = property on="Stop Cat Control" class="Bool"("DisabledEnum"=w763) -> ()  [unwired: 2 in, 2 out]
      n625 = property on="WebPages" class="Ring (strict)"("Strings []"=w773) -> ()  [unwired: 2 in, 2 out]
    }
    frame #3 {
      n626 = while {
        stop <- w776 stop-if-true
        n627 = local read "Cat Control"() -> (w774:bool)
        n628 = case shown="True" w774 {
          frame False {
          }
          frame True {
            w784 = u32 1 items=["Down/Press", "Down then Up", "Up/Release"] ("Action")
            w787 = "WebSDR" ("Such-String")
            n629 = property on="Window title" class="Str"() -> ("Value"=w779:string)  [unwired: 2 in, 2 out]
            n630 = call "Get Window RefNum.vi"("window name (\"\")"=w779) -> ("error out"=w777:errorcluster, "window refnum (NaWR)"=w778:T9)  [unwired: 7 in]
            n631 = Match Pattern(string=w779, regular expression=w787) -> (match substring=w788:string)  [unwired: 1 in, 3 out]
            n632 = for {
              N: 20 -> [_]
              tunnel: 8 -> [w911]
              tunnel: [w911] -> w783 mode=indexing
              tunnel: w784 -> [w910]
              tunnel: [w910] -> w782 mode=indexing
            }
            n633 = Equal?(x=w788, y=w787) -> (x = y?=w781:bool)
            n634 = node-c288() -> (w790:T10)  [unwired: 4 in]
            n635 = timed-loop {
              tunnel: w778 -> [w804]
              tunnel: w777 -> [w803]
              tunnel: w781 -> [w820]
              tunnel: w783 -> [w822]
              tunnel: w782 -> [w821]
              timing: w790 -> [_]
              timing-out: [_] -> w789
              tunnel: [FALSE] -> w780
              stop <- w814 stop-if-true
              n636 = local read "Downlink Freq."() -> (w806:string)
              n637 = call "Get Window Rectangle.vi"("error in (no error)"=w803, "window refnum (NaWR)"=w804) -> ("error out"=w802:errorcluster, "window rect"=w800:T2, "window refnum out"=w801:T9)  [unwired: 3 in]
              n638 = call "String Changed__ogtk.vi"("String"=w806) -> ("Changed"=w805:bool)
              n639 = local read "Truncate Left digits"() -> (w816:i32)
              n640 = Unbundle By Name(w800) -> ("left"=→"left":i16, "top"=→"top":i16, "right"=→"right":i16, "bottom"=→"bottom":i16)
              n641 = local read "Cat Control"() -> (w807:bool)
              n642 = local read "dont write"() -> (w810:bool)
              n643 = local read "OverBrowser"() -> (w792:bool)
              n644 = And(x=w805, y=w820) -> (x .and. y?=w808:bool)
              n645 = local read "MaOps"() -> (w809:bool)
              n646 = local read "Click"() -> (w793:bool)
              n647 = And(x=w807, y=w808) -> (x .and. y?=w811:bool)
              n648 = String Subset(string=w806, offset (0)=w816) -> (substring=w817:string)  [unwired: 1 in]
              n649 = And(x=w792, y=w793) -> (x .and. y?=w791:bool)
              n650 = Compound Arithmetic op=OR(w809, w811, w810) -> (w795:bool)
              n651 = And(x=w795, y=w791) -> (x .and. y?=w794:bool)
              n652 = case shown="True" w794 {
                tunnel: w801 -> [_ w838]
                tunnel: w802 -> [w824 w837]
                tunnel: [w824 w836] -> w823
                tunnel: w817 -> [_ w835]
                tunnel: w822 -> [_ w834]
                tunnel: w821 -> [_ w833]
                frame False {
                }
                frame True {
                  w831 = T5 0 items=["no dialog", "OK message", "continue or stop message", "OK message + warnings", "continue/stop + warnings"] ("type of dialog (OK msg:1)")
                  n653 = stacked-sequence {
                    seq-local: [w850 _ _] -> [_ _ w898]
                    tunnel: w838 -> [w847 _ _]
                    tunnel: w837 -> [w843 _ _]
                    tunnel: [w842 _ _] -> w836
                    tunnel: [_ _ w898] -> w832
                    tunnel: w835 -> [_ w863 _]
                    tunnel: w834 -> [_ w856 _]
                    tunnel: w833 -> [_ w855 _]
                    frame #0 {
                      n654 = call "Show Window.vi"("error in (no error)"=w843, "window refnum (NaWR)"=w847) -> ("error out"=w844:errorcluster, "window refnum out"=w846:T9)  [unwired: 4 in]
                      n655 = call "Move Window to Top.vi"("error in (no error)"=w844, "activate? (T)"=TRUE ("activate? (F)"), "window refnum (NaWR)"=w846) -> ("error out"=w845:errorcluster, "window refnum out"=w848:T9)  [unwired: 3 in]
                      n656 = call "Get Window Rectangle.vi"("error in (no error)"=w845, "window refnum (NaWR)"=w848) -> ("error out"=w842:errorcluster, "window rect"=w841:T2, "window refnum out"=w850:T9)  [unwired: 3 in]
                      n657 = local write "window rect 2"(w841) -> ()
                    }
                    frame #1 {
                      w853 = u32 1 items=["Down/Press", "Down then Up", "Up/Release"] ("Action")
                      w865 = u32 1 items=["Down/Press", "Down then Up", "Up/Release"] ("Action")
                      n658 = String To Byte Array(string=w863) -> (unsigned byte array=w852:u8[])
                      n659 = for {
                        tunnel: w852 -> [w891] mode=indexing
                        tunnel: [w890] -> w868 mode=indexing
                        tunnel: [w889] -> w867 mode=indexing
                        w889 = u32 1 items=["Down/Press", "Down then Up", "Up/Release"] ("Action")
                        n660 = Equal?(x=w891, y=u8 46 ("Extended Keaystrokes_original_control 2")) -> (x = y?=w894:bool)
                        n661 = Select(t=u8 190 ("Extended Keaystrokes_original_control 2"), s=w894, f=w891) -> (s? t:f=w890:u8)
                      }
                      n662 = Insert Into Array(array=w856, new element #1=u8 71 ("Virtual Key 2"), new element #2=w868, new element #3=u8 9 ("Extended Keaystrokes_original_control 2")) -> (w866:i32[])  [unwired: 1 in]
                      n663 = Insert Into Array(array=w855, new element #1=w853, new element #2=w867, new element #3=w865) -> (w860:u32[])  [unwired: 1 in]
                      n664 = Array Size(array=w860) -> (size(s)=w859:i32)
                      n665 = Increment(x=w859) -> (x+1=w858:i32)
                      n666 = Increment(x=w858) -> (x+1=w857:i32)
                      n667 = node-c288(i64 100 ("Period")) -> (w862:T10)  [unwired: 3 in]
                      n668 = timed-loop {
                        tunnel: w866 -> [w873] mode=indexing
                        tunnel: w860 -> [w874] mode=indexing
                        timing: w862 -> [_]
                        timing-out: [_] -> w861
                        tunnel: w857 -> [w871]
                        i -> [w872]
                        stop <- w870 stop-if-true
                        n669 = local read "OverBrowser"() -> (w869:bool)
                        n670 = case shown="True" w869 {
                          tunnel: w874 -> [_ w882]
                          tunnel: w873 -> [_ w881]
                          tunnel: w872 -> [_ w880]
                          tunnel: w871 -> [_ w879]
                          tunnel: [TRUE w877] -> w870
                          frame False {
                          }
                          frame True {
                            n671 = local read "Interrupt"() -> (w876:bool)
                            n672 = Equal?(x=w880, y=w879) -> (x = y?=w878:bool)
                            n673 = Or(x=w878, y=w876) -> (x .or. y?=w877:bool)
                            n674 = call "Simulate Keyboard.vi"("Action"=w882, "Virtual Key"=w881) -> ()  [unwired: 7 in, 1 out]
                          }
                        }
                      }
                      n675 = node-c288(w861) -> ()
                    }
                    frame #2 {
                      n676 = node-c288() -> (w897:T10)  [unwired: 4 in]
                      n677 = timed-loop {
                        shift-right: [w900] -> _
                        shift-left: FALSE ("Time has Elapsed") -> [w899]
                        timing: w897 -> [_]
                        timing-out: [_] -> w896
                        stop <- w900 stop-if-true
                        n678 = call "Elapsed Time"("Time Target (s)"=0.5, "Reset"=w899) -> ("Time has Elapsed"=w900:bool)  [unwired: 10 in, 7 out]
                      }
                      n679 = node-c288(w896) -> ()  [unwired: 1 out]
                    }
                  }
                  n680 = call "Show Window.vi"("window refnum (NaWR)"=w832) -> ("error out"=w828:errorcluster)  [unwired: 5 in, 1 out]
                  n681 = local read "FocusCheck"() -> (w825:bool)
                  n682 = Unbundle By Name(w828) -> ("status"=w826:bool)
                  n683 = call <vilib>:"Clear Errors.vi"("error in (no error)"=w828) -> ("error out"=w830:errorcluster)  [unwired: 5 in, 1 out]
                  n684 = And(x=w825, y=w826) -> (x .and. y?=w827:bool)
                  n685 = case shown="True" w827 {
                    tunnel: "There sems to be\nan issue focussing\nyour WebSDR!\n\nTry disengage and reangage" ("message") -> [_ w840]
                    frame False {
                    }
                    frame True {
                      n686 = One Button Dialog(message=w840, button name ("OK")="Wilco") -> ()  [unwired: 1 out]
                    }
                  }
                  n687 = call <vilib>:"Simple Error Handler.vi"("type of dialog (OK msg:1)"=w831, "error in (no error)"=w830) -> ()  [unwired: 3 in, 5 out]
                }
              }
              "error out" <- w823
              n688 = local read "StopCatProgramatically"() -> (w812:bool)
              n689 = property on="kill" class="Bool (strict)"() -> ("Value"=w818:bool)  [unwired: 2 in, 2 out]
              n690 = Or(x="Stop Cat Control", y=w818) -> (x .or. y?=w815:bool)
              n691 = Or(x=w812, y=w815) -> (x .or. y?=w814:bool)
            }
            n692 = node-c288(w789) -> ()  [unwired: 1 out]
            n693 = local write "StopCatProgramatically"(w780) -> ()
          }
        }
        n694 = property on="kill" class="Bool (strict)"() -> ("Value"=w776:bool)  [unwired: 2 in, 2 out]
        n695 = Wait (ms)(milliseconds to wait=u32 250) -> ()  [unwired: 1 out]
      }
    }
    frame #4 {
      n696 = while {
        tunnel: errorcluster {"status"=FALSE, "code"=0, "source"=""} ("error in (no error)") -> [w925]
        tunnel: [TRUE] -> w912
        stop <- w923 stop-if-true
        n697 = local read "Numeric"() -> (w917:i32)
        n698 = Compound Arithmetic op=AND("slave1Killed", "slave3Killed", "slave4Killed") -> ()  [unwired: 1 out]
        n699 = control-ref of="iterCompleted"() -> (w922:refnum<vi>)
        n700 = property on="iterCompleted" class="Bool (strict)"("Value"="slave1Killed") -> ()  [unwired: 2 in, 2 out]
        n701 = local write "iterCompleted"("slave1Killed") -> ()
        n702 = call "Marquee.vi"("Indicator or ctrl to look up value change"=w922, "Iteration"=w917, "error in (no error)"=w925, "Text"="Closing WebSDR Cat-Control....") -> ("shutdown"=w924:bool)  [unwired: 6 in, 1 out]
        "shutdown in" <- w924
        n703 = Or(x=w924, y="slave1Killed") -> (x .or. y?=w923:bool)
        n704 = Wait (ms)(milliseconds to wait=u32 1000) -> ()  [unwired: 1 out]
      }
      n705 = local write "Radio Mode"(TRUE ("Radio Mode")) -> ()
      n706 = local write "slave1Killed"(TRUE ("slave1Killed")) -> ()
      n707 = property on="iterCompleted" class="Bool (strict)"("Value"=FALSE ("iterCompleted")) -> ()  [unwired: 2 in, 2 out]
      n708 = Stop(stop? (T)=w912) -> ()
    }
  }
  n709 = while {
    shift-right: [w939] -> _
    shift-left: _ -> [w940]
    tunnel: [TRUE] -> w13
    stop <- "kill" stop-if-true
    w935 = u32 16860 ("Text.Text Colors:Text Color")
    w931 = T13 0 items=["Beide", "String-Anfang", "String-Ende"] ("location (both)")
    n710 = Wait (ms)(milliseconds to wait=u32 500) -> ()  [unwired: 1 out]
    n711 = local read "data"() -> (w932:string)
    n712 = Match Pattern(string=w932, regular expression="AZ" ("Regulärer Ausdruck")) -> (after substring=w950:string)  [unwired: 1 in, 3 out]
    n713 = Match Pattern(string=w932, regular expression="SN\"" ("Regulärer Ausdruck")) -> (after substring=w953:string)  [unwired: 1 in, 3 out]
    n714 = Match Pattern(string=w932, regular expression="DN" ("Regulärer Ausdruck")) -> (after substring=w952:string)  [unwired: 1 in, 3 out]
    n715 = Match Pattern(string=w932, regular expression="DM" ("Regulärer Ausdruck")) -> (after substring=w956:string)  [unwired: 1 in, 3 out]
    n716 = Match Pattern(string=w950, regular expression="EL" ("Regulärer Ausdruck")) -> (before substring=w960:string, after substring=w951:string)  [unwired: 1 in, 2 out]
    n717 = Match Pattern(string=w953, regular expression="\" " ("Regulärer Ausdruck")) -> (before substring=w962:string)  [unwired: 1 in, 3 out]
    n718 = Match Pattern(string=w952, regular expression=" " ("Regulärer Ausdruck")) -> (before substring=w955:string)  [unwired: 1 in, 3 out]
    n719 = Match Pattern(string=w956, regular expression=" " ("Regulärer Ausdruck")) -> (before substring=w957:string)  [unwired: 1 in, 3 out]
    n720 = local write "Type of DN"(w957) -> ()
    n721 = Match Pattern(string=w951, regular expression="DN" ("Regulärer Ausdruck")) -> (before substring=w958:string)  [unwired: 1 in, 3 out]
    n722 = call <vilib>:"Trim Whitespace.vi"("string"=w960, "location (both)"=w931) -> ("trimmed string"=→"Azimuth":string)
    n723 = call <vilib>:"Trim Whitespace.vi"("string"=w958, "location (both)"=w931) -> ("trimmed string"=→"Elevation":string)
    n724 = call <vilib>:"Trim Whitespace.vi"("string"=w962, "location (both)"=w931) -> ("trimmed string"=→"Satellite Name":string)
    n725 = case shown="True" "Radio Mode" {
      tunnel: w955 -> [w978 _]
      tunnel: [w976 w995] -> w939
      tunnel: ["Radio Automatic mode" "Radio Manual mode"] -> w954
      tunnel: w940 -> [_ w990]
      frame False {
        n726 = Fract/Exp String To Number(use system decimal point (T)=FALSE, string=w978) -> (number=w974:dbl)  [unwired: 2 in, 1 out]
        n727 = Divide(x=w974, y=1000.0) -> (x/y=w973:dbl)
        n728 = property on="Mode" class="Str"("Text.TextColor"=u32 16711680) -> ()  [unwired: 2 in, 2 out]
        n729 = property on="ManualLatch" class="Bool"("Visible"=FALSE ("Sichtbar")) -> ()  [unwired: 2 in, 2 out]
        n730 = property on="Downlink Freq." class="Str"("Visible"=TRUE) -> ()  [unwired: 2 in, 2 out]
        n731 = property on="Downlink Freq. Man." class="DigNum (strict)"("Visible"=FALSE) -> ()  [unwired: 2 in, 2 out]
        n732 = local read "Downlink corr."() -> (w970:dbl)
        n733 = Add(x=w973, y=w970) -> (x+y=w968:dbl)
        n734 = local write "dont write"(TRUE ("dont write")) -> ()
        n735 = Number To Fractional String(use system decimal point (T)=FALSE, number=w968, precision (6)=i16 2) -> (F-format string=w976:string)  [unwired: 1 in]
      }
      frame True {
        n736 = local read "Downlink corr."() -> (w992:dbl)
        n737 = property on="Mode" class="Str"("Text.TextColor"=u32 6618880) -> ()  [unwired: 2 in, 2 out]
        n738 = property on="ManualLatch" class="Bool"("Visible"=TRUE ("Sichtbar")) -> ()  [unwired: 2 in, 2 out]
        n739 = property on="Downlink Freq. Man." class="DigNum (strict)"("Visible"=TRUE) -> ()  [unwired: 2 in, 2 out]
        n740 = property on="Downlink Freq." class="Str"("Visible"=FALSE) -> ()  [unwired: 2 in, 2 out]
        n741 = Add(x="Downlink Freq. Man.", y=w992) -> (x+y=w986:dbl)
        n742 = Number To Fractional String(use system decimal point (T)=FALSE, number=w986, precision (6)=i16 2) -> (F-format string=w985:string)  [unwired: 1 in]
        n743 = case shown="False" "ManualLatch" {
          tunnel: [w1000 w1002] -> w995
          tunnel: w985 -> [_ w1002]
          tunnel: w990 -> [w1000 _]
          tunnel: [FALSE TRUE] -> w983
          frame False {
          }
          frame True {
          }
        }
        "MaOps" <- w983
        n744 = local write "dont write"(FALSE ("dont write")) -> ()
      }
    }
    "Mode" <- w954
    "Downlink Freq." <- w939
    n745 = property on="processes Box" class="CmbBox"() -> ("DisabledEnum"=w930:T6)  [unwired: 2 in, 2 out]
    n746 = call "I8 Changed__ogtk.vi"("I8"=w930) -> ("Changed"=w929:bool)
    n747 = call "Elapsed Time3"("Reset"=w929) -> ("Time has Elapsed"=w933:bool)  [unwired: 11 in, 7 out]
    n748 = case shown="True" w933 {
      frame False {
      }
      frame True {
        w966 = T6."Disabled and Grayed Out" ("Disabled")
        n749 = property on="FocusWebSDR" class="Bool"("DisabledEnum"=w966) -> ()  [unwired: 2 in, 2 out]
        n750 = property on="AddWebSDR" class="Bool"("DisabledEnum"=w966) -> ()  [unwired: 2 in, 2 out]
        n751 = property on="processes Box" class="CmbBox"("DisabledEnum"=w966) -> ()  [unwired: 2 in, 2 out]
      }
    }
    n752 = control-ref of="WebSDR Location / Name"() -> (w938:refnum<vi>)
    n753 = control-ref of="Truncate digits"() -> (w937:refnum<vi>)
    n754 = control-ref of="WebSDR URL"() -> (w936:refnum<vi>)
    n755 = property on="Property Node" class="Str"(reference=w938, "Text.TextColor"=w935) -> ()  [unwired: 1 in, 2 out]
    n756 = property on="Property Node" class="Str"(reference=w937, "Text.TextColor"=w935) -> ()  [unwired: 1 in, 2 out]
    n757 = property on="Property Node" class="Str"(reference=w936, "Text.TextColor"=w935) -> ()  [unwired: 1 in, 2 out]
  }
  n758 = local write "slave4Killed"(w13) -> ()
  "Title 2" <- "WebSDR Cat Control" ("Title 2")
  "Title 3" <- "WebSDR Cat Control" ("Title 3")
